vi "SO2 43i Serial Data Recording & DECADEv4.0.vi"() -> ()   [LabVIEW 2014]
uses:
  <vilib>/Instr/_visa.llb/VISA Set IO Buffer Mask.ctl
  <vilib>/Platform/TimedLoop/XDataNode/timing_clust.ctl
  <vilib>/Platform/TimedLoop/XDataNode/nitl_modes.ctl
  <vilib>/Platform/TimedLoop/XDataNode/wakeup.ctl
  C:/Program Files (x86)/National Instruments/LabVIEW 2014/examples/Data Communication/Network Streams/Simple Network Streams/support/Network Stream Command.ctl
  <vilib>/Utility/error.llb/whitespace.ctl
  <vilib>/Instr/_visa.llb/VISA Configure Serial Port (Instr).vi
  <vilib>/Utility/file.llb/Read From Spreadsheet File (string).vi
  <vilib>/Utility/tcp.llb/UDP Multicast Write-Only Open.vi
  <vilib>/platform/TimedLoop/XDataNode/XDataNode.xnode
  <vilib>/Platform/TimedLoop/XDataNode/XDNodeRunTimeDep.lvlib
  <vilib>/ptbypt/NI_PtbyPt.lvlib
panel:
  out "local\ndummy":bool
  out "cal gas cylinder conc":dbl=500.0 format="%.4g"
  out "calcon save to file":bool
  out "ev8 zero interval":i32=600
  out "Auto Zeroing":bool
  out "Simulate MOCCA Conc":dbl
  out "MOCCA window delay time (sec)":i32=30
  out "MOCCA SO2 Limit":i32=800
  out "SO2 Inflight MOCCA Alarm\n(default = OFF)":bool
  out "ev8 user set time":i32=60
  out "Mean Cal Offset":dbl
  out "Mean Cal\n(default = ON)":bool=TRUE
  out "Default file name":string
  out "Stop File Write":bool
  out "error out 4":errorcluster
  out "V6":bool
  out "V8":bool
  out "V9":bool
  out "error out 2":errorcluster
  in  "MFC_2 SLPM set value":dbl
  out "Value Read 2":string
  out "status 2":bool
  out "MFC 2":dbl[](array[numeric])
  in  "VISA resource name 3":refnum<visa-resource-name>="ASRL4::INSTR"
  in  "timeout (10sec) 3":u32=3000
  out "error out 3":errorcluster
  in  "MFC_3 SLPM set value":dbl=2.0
  out "Value Read 3":string
  out "status":bool
  out "MFC 3":dbl[](array[numeric])
  in  "VISA resource name 2":refnum<visa-resource-name>="ASRL5::INSTR"
  in  "timeout (10sec) 2":u32=3000
  out "Data Array UDP":string[](array[string])
  out "Slope":dbl=1.1
  out "Zero":dbl
  out "Simulate TWA Conc":dbl
  out "8hr_TWA_limit":i32=490
  out "10mins_STEL_limit":i32=800
  out "Simulate STEL Conc":dbl
  out "Simulate\nconc":bool
  out "q_size 2":i32
  out "8hr_so2_avg 2":dbl=1.0
  out "10min_so2_avg":dbl=1.0
  out "q_size":i32
  in  "Clear Display\nErrors":bool
  out "Data Processing":bool
  out "Serial Visa Error":errorcluster
  out "SEPTIC TCP Error Out":errorcluster
  out "TCP packet\nSend to SEPTIC":bool
  out "UDP Time Stamp Offset":i32=1
  out "Data Array TCP":string[](array[string])
  out "UDP packet \nstatus":bool
  out "UDP_Out_Error":errorcluster
  out "FISH TCP Error Out":errorcluster
  out "TCP packet\nSend to FISH":bool
  out "TCP Binary Packet":string
  out "Scan from String Error Counter\nfrom process loop":i32
  out "Read Error Counter\nfrom process loop":i32
  in  "milliseconds to wait":u32=330
  in  "ID":string="µ"
  in  "VISA resource name":refnum<visa-resource-name>="ASRL6::INSTR"
  out "Data In Array":string[](array[string])
  out "UDP_ASCII_Out":string
  out "UDP_Pack_num":u32
  out "Flight Number":string
  in  "dummy":string="00"
  out "Data String":string
  out "Internal packet":string[](array[string])
  out "RAW DATA":string
  in  "stop":bool
  out "Time taken history":u32(graph)
  out "Max Acq Time diff":u32
  out "Acq Time":u32
  out "Number of Send & Read Error\nfrom Acquire Loop":i32
  out "Command In":string
  # "SO2_conc"
  # "PMT_Volt"
  # "Lamp_Volt"
  # "Lamp_Intensity_Hz"
  # "Internal_Temp_degC"
  # "Reaction_Chamber_Temp_degC"
  # "Reaction_Chamber_Press_mmHg"
  # "Sample_Flow_litre_per_minute"
  # "Flag"
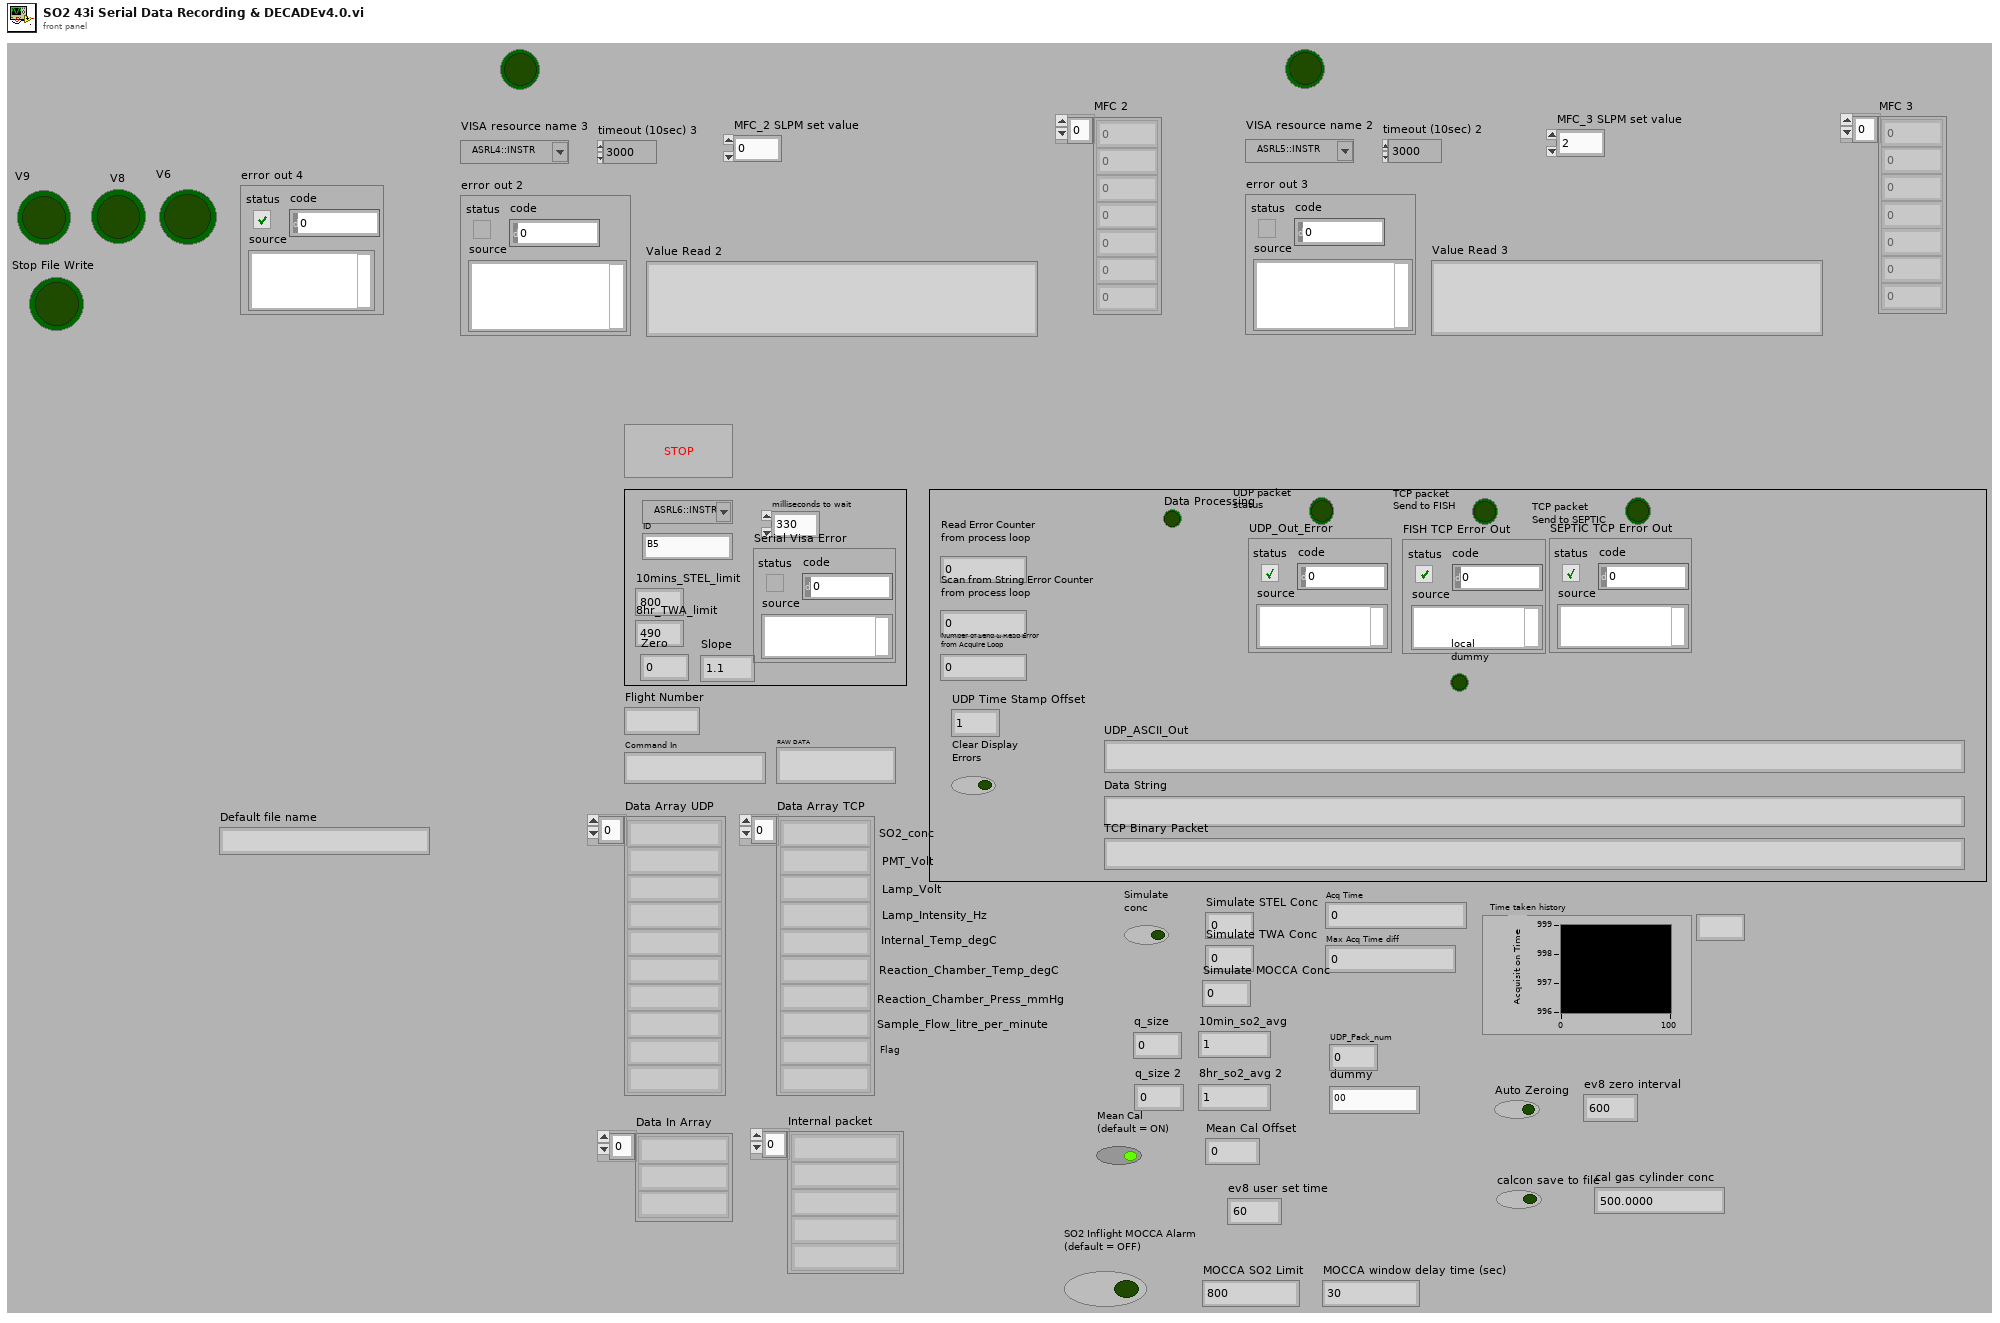
[diagram p1: front panel]
types:
  T1 = typedef "VISA Set IO Buffer Mask.ctl" = u16
  T2 = enum16{"open", "replace", "create", "open or create", "replace or create", "replace or create with confirmation"}
  T3 = typedef "Network Stream Command.ctl" = cluster{"Message":string, "Message Data":variant}
  T4 = typedef "XDNodeRunTimeDep.lvlib/timing_clust.ctl" = cluster{"Expected End [f-1]":u64, "Actual End [f-1]":u64, "Finished Late? [f-1]":bool, "Expected End [i-1]":u64, "Actual End [i-1]":u64, "Finished Late? [i-1]":bool, "Expected Start [i]":u64, "Actual Start [i]":u64, "Expected Start [f]":u64, "Actual Start [f]":u64, "Source Name":string, "Structure Name":string, "Period":i64, "Deadline":i64, "Offset":i64, "Start":i64, "Priority":i32, "Timeout":i32, "Mode":T5, "Wakeup Reason":T6, "Error":errorcluster, "Source Type":string, "Secondary Source Type":string, "Global End Time":u64, "Global Start Time":u64, "Frame Duration":u64, "Iteration Duration":u64, "Assigned CPU":i32, "I/O Scan Engine Mode":u32}
  T5 = typedef "XDNodeRunTimeDep.lvlib/nitl_modes.ctl" = enum32{"No Change", "Process missed periods, maintain original phase", "Discard missed periods, maintain original phase", "Process missed periods, ignore original phase", "Discard missed periods, ignore original phase"}
  T6 = typedef "XDNodeRunTimeDep.lvlib/wakeup.ctl" = enum32{"Normal", "Aborted", "Asynchronous wakeup", "Timing source error", "Timed loop error", "Timeout"}
  T7 = typedef "whitespace.ctl" = u16
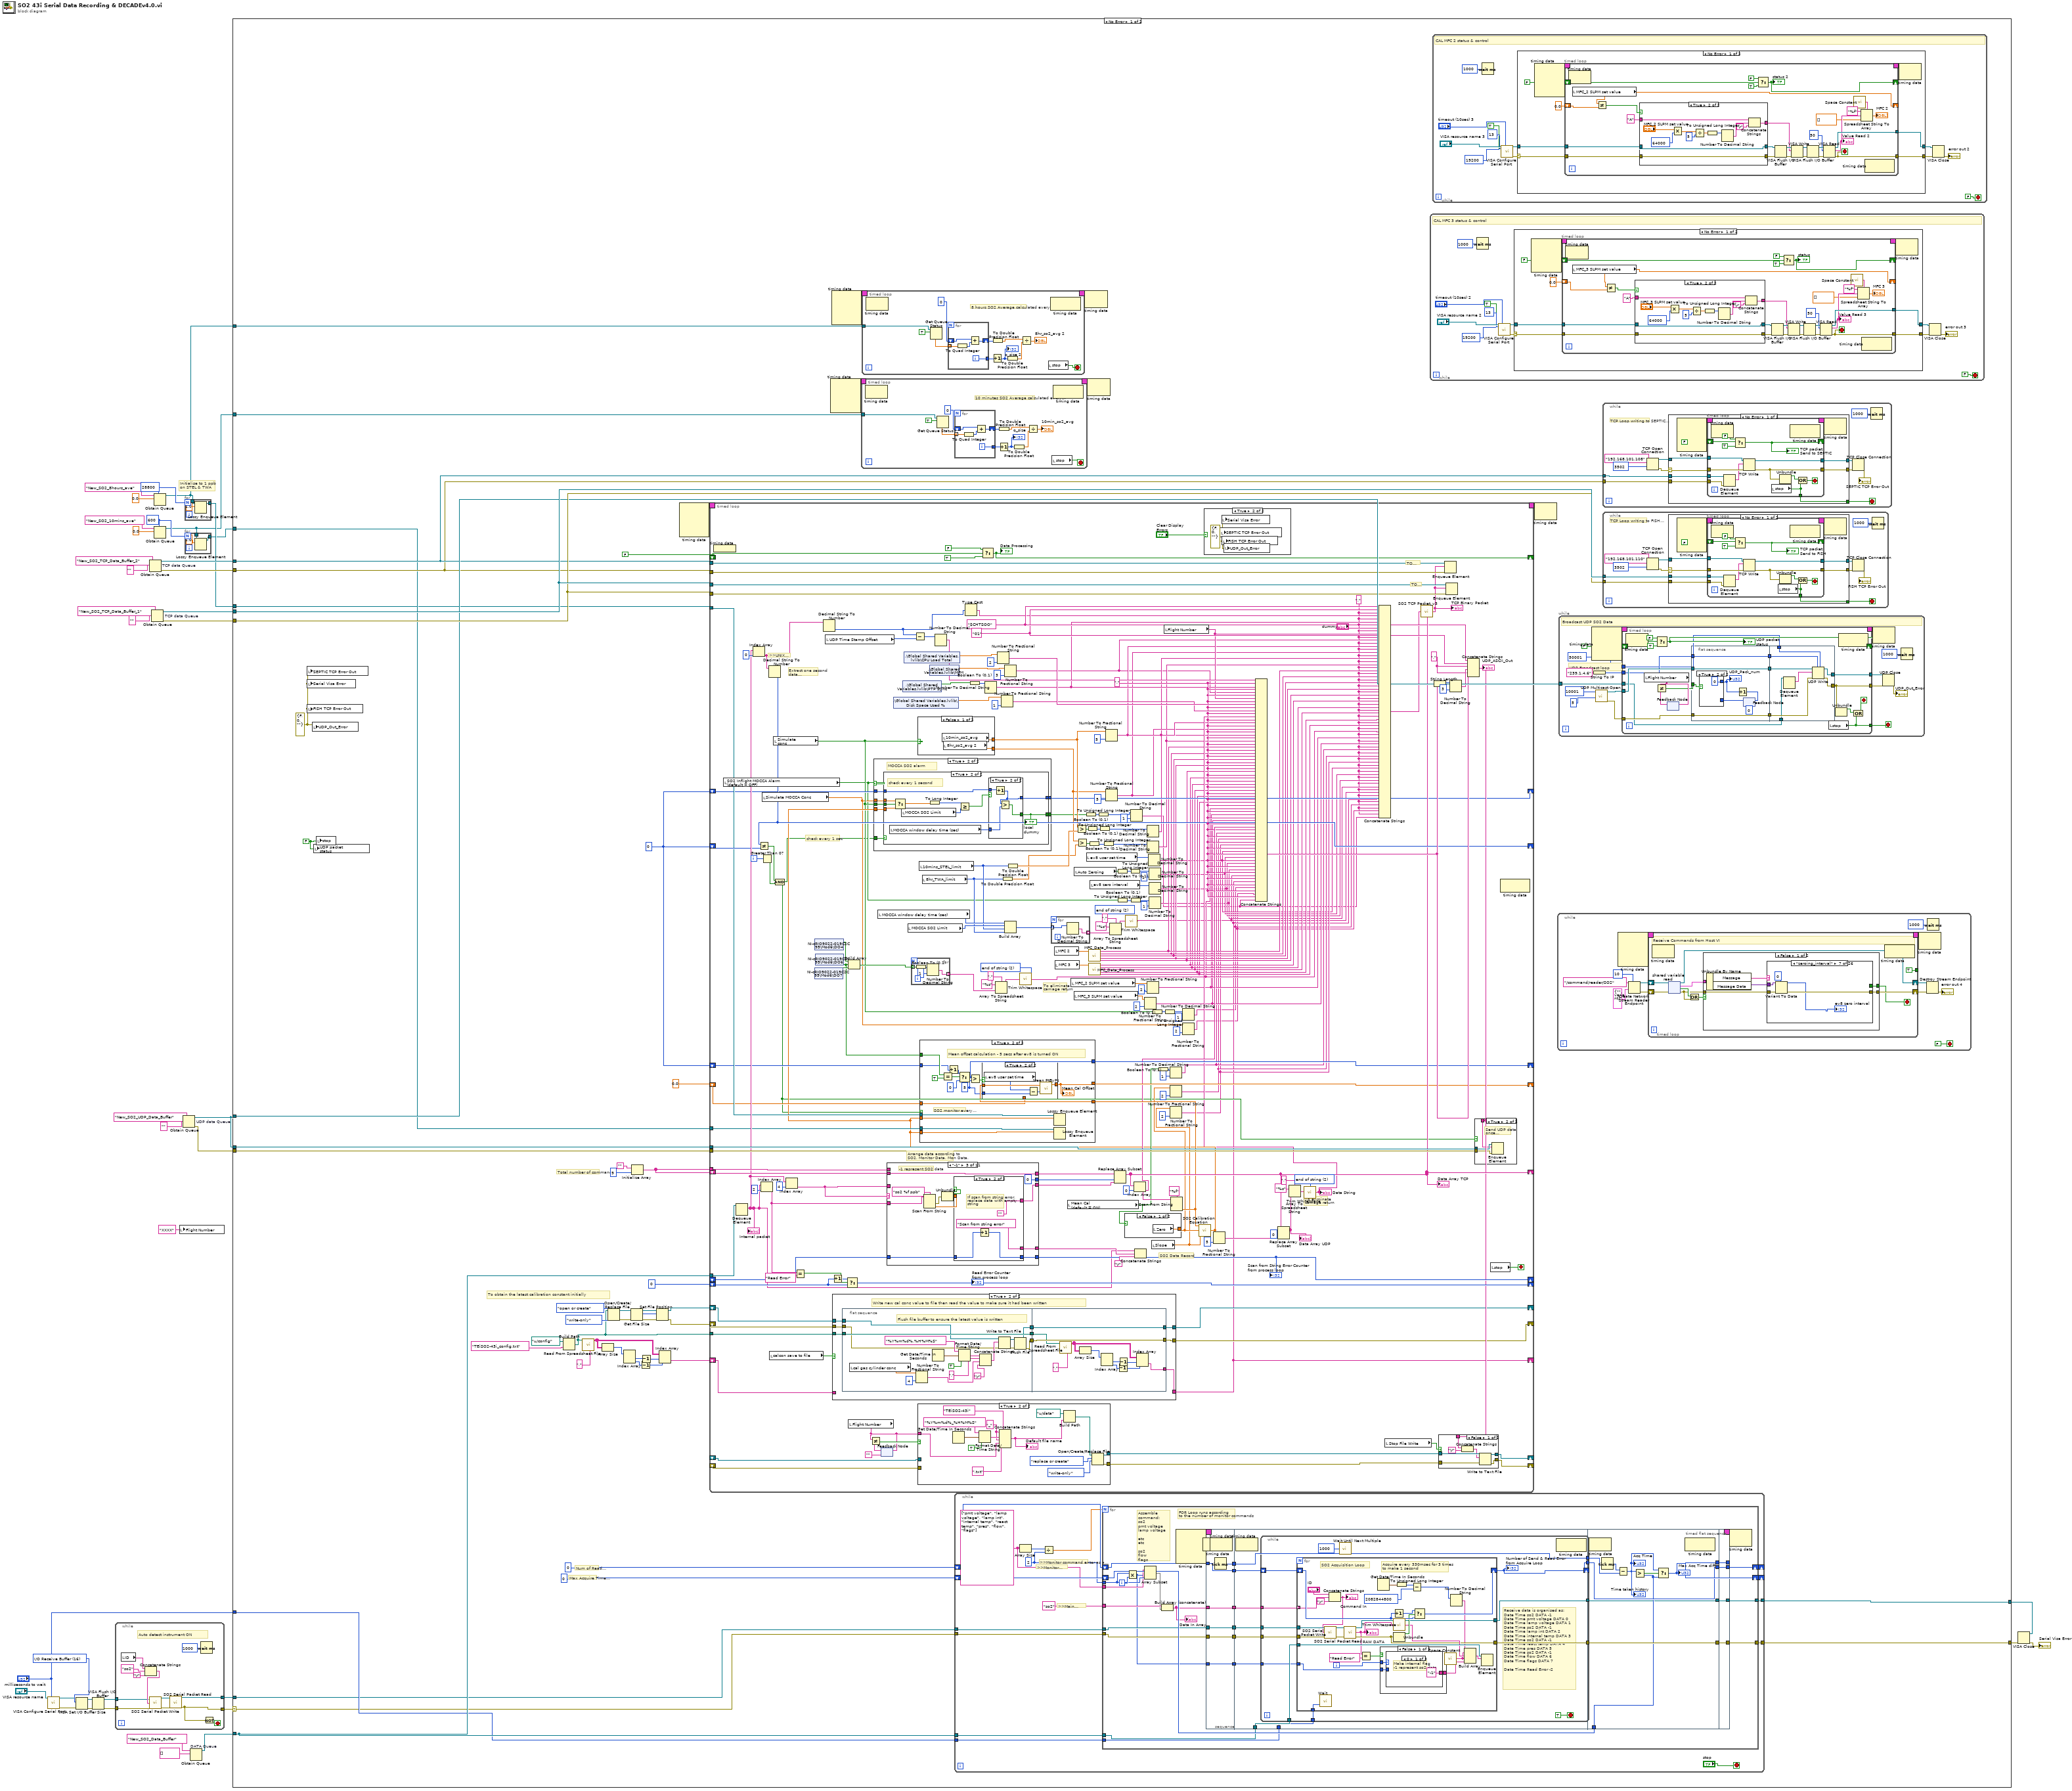
[diagram p0: block diagram]
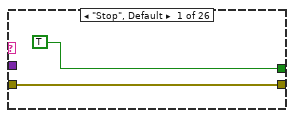
[diagram p2: hidden frame]
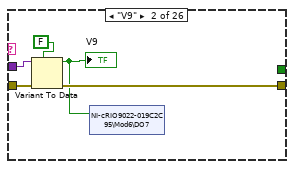
[diagram p3: hidden frame]
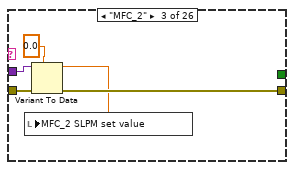
[diagram p4: hidden frame]
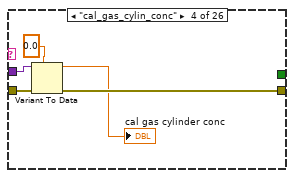
[diagram p5: hidden frame]
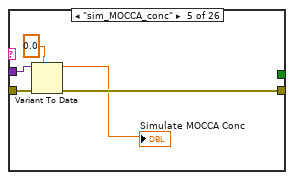
[diagram p6: hidden frame]
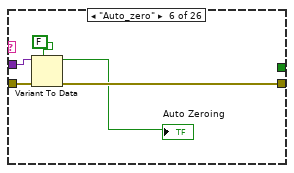
[diagram p7: hidden frame]
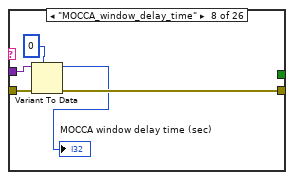
[diagram p8: hidden frame]
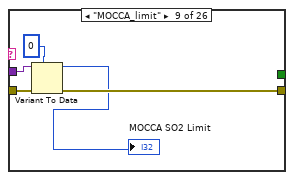
[diagram p9: hidden frame]
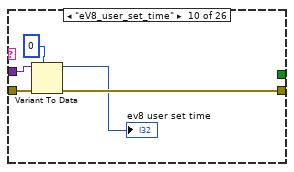
[diagram p10: hidden frame]
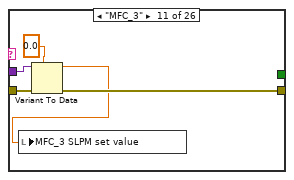
[diagram p11: hidden frame]
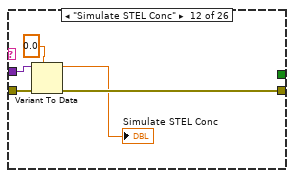
[diagram p12: hidden frame]
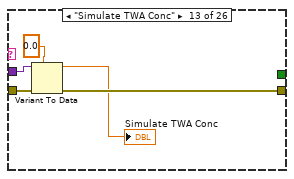
[diagram p13: hidden frame]
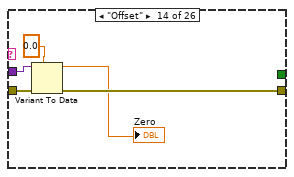
[diagram p14: hidden frame]
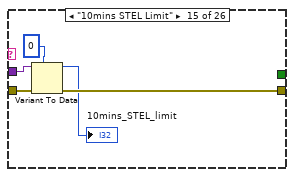
[diagram p15: hidden frame]
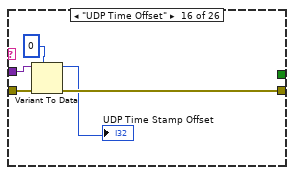
[diagram p16: hidden frame]
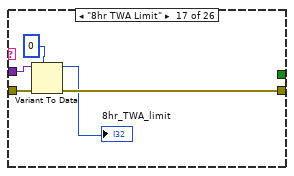
[diagram p17: hidden frame]
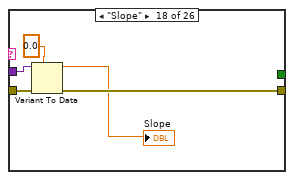
[diagram p18: hidden frame]
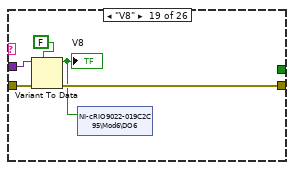
[diagram p19: hidden frame]
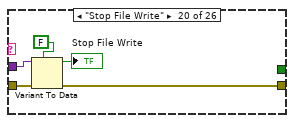
[diagram p20: hidden frame]
diagram:
  w9 = T1 16 items=["I/O Receive Buffer"=16, "I/O Transmit Buffer"=32, "I/O Receive and Transmit Buffer"=48] ("Mask")
  w16 = 28800 ("max queue size (-1, unlimited)")
  w13 = 600 ("max queue size (-1, unlimited)")
  # "Initialise to 1 ppb\non STEL & TWA"
  n1 = call-poly "VISA Configure Serial Port"("VISA resource name"="VISA resource name", "timeout (10sec)"="milliseconds to wait") -> ("VISA resource name out"=w8:refnum<visa-resource-name>, "error out"=w7:errorcluster)  [unwired: 12 in]
  n2 = VISA Set I/O Buffer Size(VISA resource name=w8, mask (16)=w9, error in (no error)=w7) -> (VISA resource name out=w2:refnum<visa-resource-name>, error out=w10:errorcluster)  [unwired: 1 in]
  n3 = VISA Flush I/O Buffer(VISA resource name=w2, error in (no error)=w10) -> (VISA resource name out=w6:refnum<visa-resource-name>, error out=w5:errorcluster)  [unwired: 1 in]
  n4 = while {
    tunnel: w6 -> [w45]
    tunnel: w5 -> [w44]
    tunnel: [w43] -> w4
    tunnel: [w42] -> w3
    stop <- w41 stop-if-true
    # "Auto detect instrument ON"
    n5 = local read "ID"() -> (w46:string)
    n6 = Concatenate Strings(w46, "so2" ("string"), "\r") -> (w49:string)
    n7 = call "SO2 Serial Packet Write.vi"("VISA resource name In"=w45, "Data in"=w49, "error in (no error)"=w44) -> ("VISA resource name Out"=w51:refnum<visa-resource-name>, "error out"=w50:errorcluster)  [unwired: 11 in]
    n8 = call "SO2 Serial Packet Read.vi"("VISA resource In"=w51, "error in"=w50) -> ("VISA resource Out"=w42:refnum<visa-resource-name>, "error out"=w43:errorcluster)  [unwired: 11 in, 1 out]
    n9 = Wait (ms)(milliseconds to wait=u32 1000) -> ()  [unwired: 1 out]
    n10 = Not(x=w43) -> (.not. x?=w41:bool)
  }
  n11 = Obtain Queue "TCP data Queue"(name (unnamed)="New_SO2_TCP_Data_Buffer_2", element data type="") -> (queue out=w23:refnum<queue>, error out=w22:errorcluster)  [unwired: 3 in, 1 out]
  n12 = Obtain Queue "TCP data Queue"(name (unnamed)="New_SO2_TCP_Data_Buffer_1", element data type="") -> (queue out=w31:refnum<queue>, error out=w30:errorcluster)  [unwired: 3 in, 1 out]
  n13 = Obtain Queue(max queue size (-1, unlimited)=w16, name (unnamed)="New_SO2_8hours_ave", element data type=0.0 ("index")) -> (queue out=w15:refnum<queue>)  [unwired: 2 in, 2 out]
  n14 = Obtain Queue(max queue size (-1, unlimited)=w13, name (unnamed)="New_SO2_10mins_ave", element data type=0.0 ("index")) -> (queue out=w12:refnum<queue>)  [unwired: 2 in, 2 out]
  n15 = local write "Flight Number"("XXXX" ("Flight Number")) -> ()
  n16 = Obtain Queue "UDP data Queue"(name (unnamed)="New_SO2_UDP_Data_Buffer", element data type="") -> (queue out=w26:refnum<queue>, error out=w27:errorcluster)  [unwired: 3 in, 1 out]
  n17 = for {
    N: w16 -> [_]
    tunnel: w15 -> [w55]
    tunnel: [w54] -> w14
    n18 = Lossy Enqueue Element(queue=w55, element=1.0) -> (queue out=w54:refnum<queue>)  [unwired: 1 in, 3 out]
  }
  n19 = for {
    N: w13 -> [_]
    tunnel: [w58] -> w11
    tunnel: w12 -> [w56]
    n20 = Lossy Enqueue Element(queue=w56, element=1.0) -> (queue out=w58:refnum<queue>)  [unwired: 1 in, 3 out]
  }
  n21 = Obtain Queue "DATA Queue"(name (unnamed)="New_SO2_Data_Buffer", element data type=string[] []) -> (queue out=w38:refnum<queue>)  [unwired: 3 in, 2 out]
  n22 = case shown="No Error" w4 {
    selector: w4 -> [w81 w1283]
    tunnel: [w112 w1283] -> w35
    tunnel: [w111 w1282] -> w36
    tunnel: w38 -> [w108 _]
    tunnel: w3 -> [w82 w1282]
    tunnel: w31 -> [w100 _]
    tunnel: w30 -> [w99 _]
    tunnel: w26 -> [w98 _]
    tunnel: w27 -> [w97 _]
    tunnel: w26 -> [w96 _]
    tunnel: w23 -> [w95 _]
    tunnel: w22 -> [w94 _]
    tunnel: "milliseconds to wait" -> [w93 _]
    tunnel: w12 -> [w90 _]
    tunnel: w15 -> [w89 _]
    tunnel: w11 -> [w88 _]
    tunnel: w14 -> [w87 _]
    frame No Error {
      w79 = 0
      w91 = errorcluster {"status"=FALSE, "code"=0, "source"=""} ("UDP Error Out")
      w102 = 0
      w101 = FALSE ("stop")
      # "To obtain the latest calibration constant initially"
      # "Max Acquire Time Diff"
      # "Num of Read Error"
      # "Total number of commands"
      n23 = local write "SEPTIC TCP Error Out"(w91) -> ()
      n24 = local write "Serial Visa Error"(w91) -> ()
      n25 = local write "FISH TCP Error Out"(w91) -> ()
      n26 = local write "UDP_Out_Error"(w91) -> ()
      n27 = local write "UDP packet \nstatus"(w101) -> ()
      n28 = local write "stop"(w101) -> ()
      n29 = Build Path(base path=path "u:/config", name or relative path="TEiSO2-43i_config.txt" ("string")) -> (appended path=w61:path)
      n30 = call-poly <vilib>:"Read From Spreadsheet File.vi"("delimiter (\\t)"="," ("delimiter (\\t)"), "file path (dialog if empty)"=w61) -> ("all rows"=w70:string[][])  [unwired: 5 in, 4 out]
      n31 = Array Size(array=w70) -> (size(s)=w71:i32[])
      n32 = Open/Create/Replace File(file path (use dialog)=w61, operation (0:open)=T2."open or create", access (0:read/write)=enum16{"read/write", "read-only", "write-only"}."write-only") -> (refnum out=w63:refnum<file>, error out=w64:errorcluster)  [unwired: 3 in, 1 out]
      n33 = Index Array(array=w71) -> (element #1=w75:i32, element #2=w73:i32)  [unwired: 2 in]
      n34 = Get File Size(file=w63, error in=w64) -> (refnum out=w65:refnum<file>, size (in bytes)=w67:i64, 0:w66:errorcluster)
      n35 = Initialize Array("", 9) -> (w103:string[])
      n36 = Decrement(x=w73) -> (x-1=w72:i32)
      n37 = Decrement(x=w75) -> (x-1=w74:i32)
      n38 = Set File Position(offset (in bytes) (0)=w67, refnum=w65, error in=w66) -> (refnum out=w60:refnum<file>, error out=w59:errorcluster)  [unwired: 1 in]
      n39 = Index Array(array=w70, index (row)=w74, index (col)=w72) -> (element=w69:string)
      n40 = node-c288() -> (w110:T4)  [unwired: 4 in]
      n41 = timed-loop {
        timing: w110 -> [_]
        timing-out: [_] -> w109
        tunnel: w108 -> [w941]
        shift-right: [w873] -> _
        shift-left: w103 -> [w931]
        shift-right: [w922] -> _
        shift-left: w102 -> [w919]
        tunnel: w103 -> [w921]
        shift-right: [w917] -> _
        shift-left: w102 -> [w918]
        tunnel: w100 -> [w915]
        tunnel: w99 -> [w914]
        tunnel: w98 -> [w913]
        tunnel: w97 -> [w912]
        shift-right: [w904] -> _
        shift-left: w79 -> [w907]
        tunnel: w95 -> [w903]
        tunnel: w94 -> [w902]
        shift-right: [w895] -> _
        shift-left: FALSE -> [w898]
        tunnel: w88 -> [w892]
        tunnel: w87 -> [w891]
        shift-right: [w860] -> _
        shift-left: _ -> [w862]
        shift-right: [w859] -> _
        shift-left: _ -> [w861]
        shift-right: [w829] -> _
        shift-left: w79 -> [w831]
        shift-right: [w827] -> _
        shift-left: 0.0 -> [w828]
        shift-right: [w817] -> _
        shift-left: w79 -> [w818]
        tunnel: w61 -> [w794]
        shift-right: [w744] -> _
        shift-left: w69 -> [w793]
        shift-right: [w784] -> _
        shift-left: w60 -> [w785]
        shift-right: [w782] -> _
        shift-left: w59 -> [w783]
        i -> [w905]
        stop <- w939 stop-if-true
        w741 = ","
        (unwired) i16 1 ("width (-)")
        (unwired) T7 2 items=["both", "start of string", "end of string"] ("location (both)")
        w837 = T7 2 items=["both", "start of string", "end of string"] ("location (both)")
        w927 = T7 2 items=["both", "start of string", "end of string"] ("location (both)")
        w787 = ","
        w777 = "01"
        w933 = ","
        w778 = "$CHTSOO"
        # "check every 1 sec"
        # "To eliminate\ncarriage return"
        # "TO SEPTIC"
        # "TO FISH"
        # "Extract one second data\nfor UDP sending"
        # "Arrange data according to\nSO2, Monitor Data, Mon Data,"
        # "To eliminate\ncarriage return"
        # ">>UNIX TIME>>"
        # "SO2 Data Record"
        n42 = node-c288() -> ()  [unwired: 1 in]
        n43 = local read "SO2 Inflight MOCCA Alarm\n(default = OFF)"() -> (w780:bool)
        n44 = Dequeue Element(queue=w941) -> (element=w910:string[])  [unwired: 2 in, 3 out]
        "Internal packet" <- w910
        n45 = Index Array(array=w910, index=0) -> (element=w909:string)
        n46 = Index Array(array=w910, index=2) -> (element=w925:string)
        n47 = Greater Than 0?(x=w905) -> (x > 0?=w908:bool)
        n48 = local read "Simulate MOCCA Conc"() -> (w788:dbl)
        n49 = Decimal String To Number(string=w909) -> (number=w904:i32)  [unwired: 2 in, 1 out]
        n50 = Not Equal?(x=w904, y=w907) -> (x != y?=w906:bool)
        n51 = local read "calcon save to file"() -> (w781:bool)
        n52 = local read "Simulate\nconc"() -> (w790:bool)
        n53 = Compound Arithmetic op=AND(w906, w908) -> (w779:bool)
        n54 = Index Array(array=w910, index=4) -> (element=w894:string)
        n55 = Equal?(x=w925, y="Read Error") -> (x = y?=w923:bool)
        n56 = shared-variable "NI-cRIO9022-019C2C95\\Mod6\\DO7"() -> (w845:bool)  [unwired: 1 in, 1 out]
        n57 = shared-variable "NI-cRIO9022-019C2C95\\Mod6\\DO4"() -> (w846:bool)  [unwired: 1 in, 1 out]
        n58 = shared-variable "NI-cRIO9022-019C2C95\\Mod6\\DO6"() -> (w832:bool)  [unwired: 1 in, 1 out]
        n59 = Decimal String To Number(string=w909) -> (number=w776:i32)  [unwired: 2 in, 1 out]
        n60 = local read "UDP Time Stamp Offset"() -> (w836:i32)
        n61 = Increment(x=w919) -> (x+1=w920:i32)
        n62 = case shown="True" w781 {
          tunnel: w794 -> [_ w953]
          tunnel: [w942 w951] -> w782
          tunnel: w793 -> [w944 _]
          tunnel: [w944 w950] -> w744
          tunnel: w785 -> [w943 w948]
          tunnel: [w943 w946] -> w784
          tunnel: w783 -> [w942 w945]
          frame False {
          }
          frame True {
            # "Write new cal conc value to file then read the value to make sure it had been written"
            n63 = flat-sequence {
              tunnel: w953 -> [w961]
              tunnel: [w956] -> w952
              tunnel: [w961] -> w949
              tunnel: w948 -> [w960]
              tunnel: [w955] -> w947
              tunnel: w945 -> [w959]
              tunnel: w952 -> [w974]
              tunnel: [w974] -> w951
              tunnel: [w973] -> w950
              tunnel: w949 -> [w972]
              tunnel: w947 -> [w971]
              tunnel: [w971] -> w946
              frame #0 {
                # "Flush file buffer to ensure the latest value is written"
                n64 = local read "cal gas cylinder conc"() -> (w954:dbl)
                n65 = Number To Fractional String(number=w954, precision (6)=i16 4) -> (F-format string=w962:string)  [unwired: 2 in]
                n66 = Get Date/Time In Seconds() -> (seconds since 1Jan1904=w969:timestamp)
                n67 = Format Date/Time String(time format string (%c)="%Y%m%d%,%H%M%S", seconds (now)=w969, UTC format=TRUE) -> (date/time string=w966:string)
                n68 = Concatenate Strings(w966, "," ("string"), w962, "\r") -> (w964:string)
                n69 = Write to Text File(file (use dialog)=w960, text=w964, error in=w959) -> (refnum out=w957:refnum<file>, error out=w958:errorcluster)  [unwired: 1 in, 1 out]
                n70 = Flush File(refnum=w957, error in=w958) -> (refnum out=w955:refnum<file>, error out=w956:errorcluster)
              }
              frame #1 {
                n71 = call-poly <vilib>:"Read From Spreadsheet File.vi"("delimiter (\\t)"="," ("delimiter (\\t)"), "file path (dialog if empty)"=w972) -> ("all rows"=w975:string[][])  [unwired: 5 in, 4 out]
                n72 = Array Size(array=w975) -> (size(s)=w976:i32[])
                n73 = Index Array(array=w976) -> (element #1=w980:i32, element #2=w978:i32)  [unwired: 2 in]
                n74 = Decrement(x=w978) -> (x-1=w977:i32)
                n75 = Decrement(x=w980) -> (x-1=w979:i32)
                n76 = Index Array(array=w975, index (row)=w979, index (col)=w977) -> (element=w973:string)
              }
            }
          }
        }
        n77 = Select(t=w920, s=w923, f=w919) -> (s? t:f=w922:i32)
        "Read Error Counter\nfrom process loop" <- w922
        n78 = Build Array(w846, w832, w845) -> (w850:bool[])
        n79 = local read "Flight Number"() -> (w863:string)
        n80 = local read "MOCCA window delay time (sec)"() -> (w799:i32)
        n81 = feedback #1("" ("Flight Number")) -> (w868:string)
        n82 = Not Equal?(x=w863, y=w868) -> (x != y?=w866:bool)
        n83 = feedback-in #1(w863) -> ()
        n84 = case shown="\"-1\"" w894 {
          tunnel: w894 -> [w1081 _ _ w1117 w1138 w1159 w1181 w1203 w1225 w1247 w1269]
          tunnel: w931 -> [w1082 _ w1096 w1118 w1139 w1160 w1182 w1204 w1226 w1248 w1270]
          tunnel: w925 -> [_ _ w1093 w1113 w1134 w1156 w1178 w1200 w1222 w1244 w1266]
          tunnel: [w1082 w1085 w1096 w1118 w1139 w1160 w1182 w1204 w1226 w1248 w1270] -> w878
          tunnel: [w1079 _ 0 ("index") w1115 w1136 w1157 w1179 w1201 w1223 w1245 w1267] -> w877
          tunnel: [_ _ w1092 w1112 w1133 w1155 w1177 w1199 w1221 w1243 w1261] -> w930
          tunnel: w921 -> [_ w1085 _ _ _ _ _ _ _ _ _]
          tunnel: w918 -> [w1077 w1084 w1089 w1109 w1130 w1150 w1173 w1194 w1217 w1238 w1260]
          tunnel: [w1077 w1084 w1088 w1108 w1129 w1149 w1172 w1193 w1216 w1237 w1259] -> w917
          tunnel: ["Internal False Flag Detected" "" w1087 w1107 w1128 w1148 w1171 w1192 w1215 w1236 w1258] -> w916
          frame "False", Default {
            n85 = Decimal String To Number(string=w1081) -> (number=w1078:i32)  [unwired: 2 in, 1 out]
            n86 = Add(x=w1078, y=1) -> (x+y=w1079:i32)
          }
          frame "-2" {
            # "Read Error Detected\nMake all data as a space"
          }
          frame "-1" {
            # "-1 represent SO2 data"
            n87 = Scan From String(format string="so2 %f ppb", input string=w1093) -> (error out=w1091:errorcluster, output 1=w1086:dbl)  [unwired: 3 in, 2 out]
            n88 = Unbundle(w1091) -> ("status"=w1090:bool)  [unwired: 2 out]
            n89 = case shown="True" w1090 {
              tunnel: w1086 -> [w1097 _]
              tunnel: [w1101 ""] -> w1092
              tunnel: w1089 -> [w1100 w1105]
              tunnel: [w1100 w1104] -> w1088
              tunnel: ["" "Scan from string error"] -> w1087
              frame False {
                # "Extract the concentration\nvalue & fixed format"
                n90 = Number To Fractional String(number=w1097, precision (6)=i16 5) -> (F-format string=w1101:string)  [unwired: 2 in]
              }
              frame True {
                # "If scan from string error,\nreplace data with empty\nstring"
                n91 = Increment(x=w1105) -> (x+1=w1104:i32)
              }
            }
          }
          frame "0" {
            # "0 represents pmt voltage -0510 volts"
            n92 = Scan From String(format string="pmt voltage %d", input string=w1113) -> (error out=w1111:errorcluster, output 1=w1106:i32)  [unwired: 3 in, 2 out]
            n93 = Decimal String To Number(string=w1117) -> (number=w1116:i32)  [unwired: 2 in, 1 out]
            n94 = Unbundle(w1111) -> ("status"=w1110:bool)  [unwired: 2 out]
            n95 = case shown="False" w1110 {
              tunnel: w1106 -> [w1122 _]
              tunnel: [w1119 w1123] -> w1112
              tunnel: w1109 -> [w1121 w1126]
              tunnel: [w1121 w1125] -> w1108
              tunnel: ["" "Scan from string error"] -> w1107
              tunnel: [w1119 w1123] -> _
              frame False {
                # "Extract the actual value\n& fixed format"
                n96 = Number To Decimal String(number=w1122) -> (decimal integer string=w1119:string)  [unwired: 1 in]
              }
              frame True {
                w1123 = ""
                # "If scan from string error,\nreplace data with empty\nstring"
                n97 = Increment(x=w1126) -> (x+1=w1125:i32)
              }
            }
            n98 = Increment(x=w1116) -> (x+1=w1115:i32)
          }
          frame "1" {
            # "1 represents lamp voltage; lamp voltage 810 volts"
            n99 = Scan From String(format string="lamp voltage %d", input string=w1134) -> (error out=w1132:errorcluster, output 1=w1127:i32)  [unwired: 3 in, 2 out]
            n100 = Decimal String To Number(string=w1138) -> (number=w1137:i32)  [unwired: 2 in, 1 out]
            n101 = Unbundle(w1132) -> ("status"=w1131:bool)  [unwired: 2 out]
            n102 = case shown="True" w1131 {
              tunnel: w1127 -> [w1143 _]
              tunnel: [w1140 w1144] -> w1133
              tunnel: w1130 -> [w1142 w1147]
              tunnel: [w1142 w1146] -> w1129
              tunnel: ["" "Scan from string error"] -> w1128
              tunnel: [w1140 w1144] -> _
              frame False {
                # "Extract the actual value\n& fixed format"
                n103 = Number To Decimal String(number=w1143) -> (decimal integer string=w1140:string)  [unwired: 1 in]
              }
              frame True {
                w1144 = ""
                # "If scan from string error,\nreplace data with empty\nstring"
                n104 = Increment(x=w1147) -> (x+1=w1146:i32)
              }
            }
            n105 = Increment(x=w1137) -> (x+1=w1136:i32)
          }
          frame "2" {
            # "2 represents lamp intensity; lamp int 35867 Hz"
            n106 = Scan From String(format string="lamp int %d", input string=w1156) -> (error out=w1152:errorcluster, output 1=w1153:i32)  [unwired: 3 in, 2 out]
            n107 = Decimal String To Number(string=w1159) -> (number=w1158:i32)  [unwired: 2 in, 1 out]
            n108 = Unbundle(w1152) -> ("status"=w1151:bool)  [unwired: 2 out]
            n109 = case shown="True" w1151 {
              tunnel: [w1161 w1166] -> w1155
              tunnel: w1153 -> [w1165 _]
              tunnel: w1150 -> [w1164 w1169]
              tunnel: [w1164 w1168] -> w1149
              tunnel: ["" "Scan from string error"] -> w1148
              tunnel: [w1161 w1166] -> _
              frame False {
                # "Extract the actual value\n& fixed format"
                n110 = Number To Fractional String(number=w1165, precision (6)=i16 0) -> (F-format string=w1161:string)  [unwired: 2 in]
              }
              frame True {
                w1166 = ""
                # "If scan from string error,\nreplace data with empty\nstring"
                n111 = Increment(x=w1169) -> (x+1=w1168:i32)
              }
            }
            n112 = Increment(x=w1158) -> (x+1=w1157:i32)
          }
          frame "3" {
            # "3 represents internal temp; internal temp 027.2 deg C, actual 027.2"
            n113 = Scan From String(format string="%[^,], %s %f", input string=w1178) -> (error out=w1175:errorcluster, output 3=w1170:dbl)  [unwired: 7 in, 2 out]
            n114 = Decimal String To Number(string=w1181) -> (number=w1180:i32)  [unwired: 2 in, 1 out]
            n115 = Unbundle(w1175) -> ("status"=w1174:bool)  [unwired: 2 out]
            n116 = case shown="True" w1174 {
              tunnel: [w1183 w1188] -> w1177
              tunnel: w1170 -> [w1187 _]
              tunnel: w1173 -> [w1186 w1191]
              tunnel: [w1186 w1190] -> w1172
              tunnel: ["" "Scan from string error"] -> w1171
              tunnel: [w1183 w1188] -> _
              frame False {
                # "Extract the actual value\n& fixed format"
                n117 = Number To Fractional String(number=w1187, precision (6)=i16 1) -> (F-format string=w1183:string)  [unwired: 2 in]
              }
              frame True {
                w1188 = ""
                # "If scan from string error,\nreplace data with empty\nstring"
                n118 = Increment(x=w1191) -> (x+1=w1190:i32)
              }
            }
            n119 = Increment(x=w1180) -> (x+1=w1179:i32)
          }
          frame "4" {
            # "4 represents react temp; react temp 045.2 deg C"
            n120 = Scan From String(format string="react temp %f deg C", input string=w1200) -> (error out=w1196:errorcluster, output 1=w1197:dbl)  [unwired: 3 in, 2 out]
            n121 = Decimal String To Number(string=w1203) -> (number=w1202:i32)  [unwired: 2 in, 1 out]
            n122 = Unbundle(w1196) -> ("status"=w1195:bool)  [unwired: 2 out]
            n123 = case shown="False" w1195 {
              tunnel: [w1205 w1210] -> w1199
              tunnel: w1197 -> [w1209 _]
              tunnel: w1194 -> [w1208 w1213]
              tunnel: [w1208 w1212] -> w1193
              tunnel: ["" "Scan from string error"] -> w1192
              tunnel: [w1205 w1210] -> _
              frame False {
                # "Extract the actual value\n& fixed format"
                n124 = Number To Fractional String(number=w1209, precision (6)=i16 1) -> (F-format string=w1205:string)  [unwired: 2 in]
              }
              frame True {
                w1210 = ""
                # "If scan from string error,\nreplace data with empty\nstring"
                n125 = Increment(x=w1213) -> (x+1=w1212:i32)
              }
            }
            n126 = Increment(x=w1202) -> (x+1=w1201:i32)
          }
          frame "5" {
            # "5 represents chamber pressure; pres 760.0 mm Hg, actual 753.4"
            n127 = Scan From String(format string="%[^,], %s %f", input string=w1222) -> (error out=w1219:errorcluster, output 3=w1214:dbl)  [unwired: 7 in, 2 out]
            n128 = Decimal String To Number(string=w1225) -> (number=w1224:i32)  [unwired: 2 in, 1 out]
            n129 = Unbundle(w1219) -> ("status"=w1218:bool)  [unwired: 2 out]
            n130 = case shown="False" w1218 {
              tunnel: [w1227 w1232] -> w1221
              tunnel: w1214 -> [w1231 _]
              tunnel: w1217 -> [w1230 w1235]
              tunnel: [w1230 w1234] -> w1216
              tunnel: ["" "Scan from string error"] -> w1215
              tunnel: [w1227 w1232] -> _
              frame False {
                # "Extract the actual value\n& fixed format"
                n131 = Number To Fractional String(number=w1231, precision (6)=i16 1) -> (F-format string=w1227:string)  [unwired: 2 in]
              }
              frame True {
                w1232 = ""
                # "If scan from string error,\nreplace data with empty\nstring"
                n132 = Increment(x=w1235) -> (x+1=w1234:i32)
              }
            }
            n133 = Increment(x=w1224) -> (x+1=w1223:i32)
          }
          frame "6" {
            # "6 represents flow data; flow 0.503 l/m"
            n134 = Scan From String(format string="flow %f l/m", input string=w1244) -> (error out=w1240:errorcluster, output 1=w1241:dbl)  [unwired: 3 in, 2 out]
            n135 = Decimal String To Number(string=w1247) -> (number=w1246:i32)  [unwired: 2 in, 1 out]
            n136 = Unbundle(w1240) -> ("status"=w1239:bool)  [unwired: 2 out]
            n137 = case shown="True" w1239 {
              tunnel: [w1253 ""] -> w1243
              tunnel: w1241 -> [w1252 _]
              tunnel: w1238 -> [w1251 w1256]
              tunnel: [w1251 w1255] -> w1237
              tunnel: ["" "Scan from string error"] -> w1236
              frame False {
                # "Extract the actual value\n& fixed format"
                n138 = Number To Fractional String(number=w1252, precision (6)=i16 3) -> (F-format string=w1253:string)  [unwired: 2 in]
              }
              frame True {
                # "If scan from string error,\nreplace data with empty\nstring"
                n139 = Increment(x=w1256) -> (x+1=w1255:i32)
              }
            }
            n140 = Increment(x=w1246) -> (x+1=w1245:i32)
          }
          frame "7" {
            # "7 represents flags data; flags 1c100000"
            n141 = Scan From String(format string="flags %s", input string=w1266) -> (error out=w1264:errorcluster, output 1=w1262:string)  [unwired: 3 in, 2 out]
            n142 = Decimal String To Number(string=w1269) -> (number=w1268:i32)  [unwired: 2 in, 1 out]
            n143 = Unbundle(w1264) -> ("status"=w1263:bool)  [unwired: 2 out]
            n144 = case shown="False" w1263 {
              tunnel: w1262 -> [w1273 _]
              tunnel: [w1273 ""] -> w1261
              tunnel: w1260 -> [w1272 w1276]
              tunnel: [w1272 w1275] -> w1259
              tunnel: ["" "Scan from string error"] -> w1258
              frame False {
                # "Extract the actual value\n& fixed format"
              }
              frame True {
                # "If scan from string error,\nreplace data with empty\nstring"
                n145 = Increment(x=w1276) -> (x+1=w1275:i32)
              }
            }
            n146 = Increment(x=w1268) -> (x+1=w1267:i32)
          }
        }
        "Scan from String Error Counter\nfrom process loop" <- w917
        n147 = shared-variable ".\\Global Shared Variables.lvlib\\Disk Space Used %"() -> (w839:dbl)  [unwired: 1 in, 1 out]
        n148 = shared-variable ".\\Global Shared Variables.lvlib\\PTP Sync"() -> (w852:bool)  [unwired: 1 in, 1 out]
        n149 = shared-variable ".\\Global Shared Variables.lvlib\\CPU Load Total"() -> (w856:dbl)  [unwired: 1 in, 1 out]
        n150 = local read "MOCCA SO2 Limit"() -> (w798:i32)
        n151 = for {
          tunnel: w850 -> [w1020] mode=indexing
          tunnel: [w1019] -> w847 mode=indexing
          n152 = Boolean To (0,1)(Boolean=w1020) -> (0, 1=w1021:i16)
          n153 = Number To Decimal String(number=w1021, width (-)=i16 1) -> (decimal integer string=w1019:string)
        }
        n154 = Subtract(x=w776, y=w836) -> (x-y=w900:i32)
        n155 = case shown="False" w790 {
          tunnel: [w1013 w1014] -> w887
          tunnel: [w1012 w1015] -> w885
          frame False {
            n156 = local read "10min_so2_avg"() -> (w1013:dbl)
            n157 = local read "8hr_so2_avg 2"() -> (w1012:dbl)
          }
          frame True {
            # "SO2 STEL & TWA simulate"
            n158 = local read "Simulate STEL Conc"() -> (w1014:dbl)
            n159 = local read "Simulate TWA Conc"() -> (w1015:dbl)
          }
        }
        n160 = case shown="True" w866 {
          tunnel: [w1023 w1026] -> w865
          tunnel: [w1022 w1025] -> w864
          tunnel: w862 -> [w1023 _]
          tunnel: w861 -> [w1022 _]
          tunnel: w863 -> [_ w1024]
          frame False {
          }
          frame True {
            w1033 = "_" ("string")
            n161 = Get Date/Time In Seconds() -> (seconds since 1Jan1904=w1034:timestamp)
            n162 = Format Date/Time String(time format string (%c)="%Y%m%d%_%H%M%S", seconds (now)=w1034, UTC format=TRUE) -> (date/time string=w1037:string)
            n163 = Concatenate Strings("TEiSO2-43i" ("string"), w1033, w1037, w1033, w1024, ".txt" ("string")) -> (w1031:string)
            "Default file name" <- w1031
            n164 = Build Path(base path=path "u:/data", name or relative path=w1031) -> (appended path=w1027:path)
            n165 = Open/Create/Replace File(file path (use dialog)=w1027, operation (0:open)=T2."replace or create", access (0:read/write)=enum16{"read/write", "read-only", "write-only"}."write-only") -> (refnum out=w1026:refnum<file>, error out=w1025:errorcluster)  [unwired: 3 in, 1 out]
          }
        }
        n166 = local read "10mins_STEL_limit"() -> (w797:i32)
        n167 = local read "8hr_TWA_limit"() -> (w796:i32)
        n168 = shared-variable ".\\Global Shared Variables.lvlib\\MFM"() -> (w853:dbl)  [unwired: 1 in, 1 out]
        n169 = Number To Decimal String(number=w900) -> (decimal integer string=w899:string)  [unwired: 1 in]
        n170 = Type Cast(x=w776) -> (*(type *) &x=w775:string)  [unwired: 1 in]
        n171 = Boolean To (0,1)(Boolean=w852) -> (0, 1=w851:i16)
        n172 = Select(t=FALSE, s=w898, f=TRUE) -> (s? t:f=w895:bool)
        "Data Processing" <- w895
        n173 = Number To Decimal String(number=w851) -> (decimal integer string=w774:string)  [unwired: 1 in]
        n174 = Array To Spreadsheet String(delimiter (Tab)=",", array=w847, 3:"%s" ("format string")) -> (spreadsheet string=w838:string)
        n175 = Number To Fractional String(number=w856, precision (6)=i16 2) -> (F-format string=w835:string)  [unwired: 2 in]
        n176 = Number To Fractional String(number=w839, precision (6)=i16 1) -> (F-format string=w834:string)  [unwired: 2 in]
        n177 = To Double Precision Float(number=w796) -> (double precision float=w888:dbl)
        n178 = Number To Fractional String(number=w853, precision (6)=i16 3) -> (F-format string=w766:string)  [unwired: 2 in]
        n179 = Build Array(w799, w798, w797, w796) -> (w795:i32[])
        n180 = To Double Precision Float(number=w797) -> (double precision float=w889:dbl)
        n181 = call <vilib>:"Trim Whitespace.vi"("string"=w838, "location (both)"=w837) -> ("trimmed string"=w755:string)
        n182 = for {
          tunnel: w795 -> [w982] mode=indexing
          tunnel: [w983] -> w801 mode=indexing
          n183 = Number To Decimal String(number=w982) -> (decimal integer string=w983:string)  [unwired: 1 in]
        }
        n184 = local read "MFC 2"() -> (w870:dbl[])
        n185 = local read "MFC 3"() -> (w869:dbl[])
        n186 = local read "Mean Cal\n(default = ON)"() -> (w823:bool)
        n187 = local read "MFC_2 SLPM set value"() -> (w842:dbl)
        n188 = local read "MFC_3 SLPM set value"() -> (w841:dbl)
        n189 = local read "Auto Zeroing"() -> (w809:bool)
        n190 = Greater?(x=w887, y=w889) -> (0:w882:bool)
        n191 = Greater?(x=w885, y=w888) -> (0:w881:bool)
        n192 = local read "ev8 user set time"() -> (w812:i32)
        n193 = Boolean To (0,1)(Boolean=w882) -> (0, 1=w884:i16)
        n194 = Boolean To (0,1)(Boolean=w881) -> (0, 1=w883:i16)
        n195 = call "MFC_Data_Process.vi"("MFC"=w870) -> ("MFC Absolute Pressure"=w765:string, "MFC Temperature"=w764:string, "MFC Volumetric Flow"=w763:string, "MFC Mass Flow"=w762:string, "MFC Set Point"=w761:string)  [unwired: 10 in]
        n196 = call "MFC_Data_Process.vi"("MFC"=w869) -> ("MFC Absolute Pressure"=w760:string, "MFC Temperature"=w759:string, "MFC Volumetric Flow"=w758:string, "MFC Mass Flow"=w757:string, "MFC Set Point"=w756:string)  [unwired: 10 in]
        n197 = local read "ev8 zero interval"() -> (w808:i32)
        n198 = To Unsigned Long Integer(number=w884) -> (unsigned 32bit integer=w880:u32)
        n199 = To Unsigned Long Integer(number=w883) -> (unsigned 32bit integer=w879:u32)
        n200 = Number To Fractional String(number=w887, precision (6)=i16 5) -> (F-format string=w770:string)  [unwired: 2 in]
        n201 = Number To Fractional String(number=w885, precision (6)=i16 5) -> (F-format string=w769:string)  [unwired: 2 in]
        n202 = Array To Spreadsheet String(delimiter (Tab)=",", array=w801, 3:"%s" ("format string")) -> (spreadsheet string=w800:string)
        n203 = Replace Array Subset(array=w878, new element=w930, index=w877) -> (w873:string[])
        "Data Array TCP" <- w873
        n204 = Boolean To (0,1)(Boolean=w809) -> (0, 1=w811:i16)
        n205 = Boolean To (0,1)(Boolean=w780) -> (0, 1=w807:i16)
        n206 = case shown="False" w823 {
          tunnel: [w1016 w1017] -> w820
          frame False {
            n207 = local read "Zero"() -> (w1016:dbl)
          }
          frame True {
            n208 = local read "Mean Cal Offset"() -> (w1017:dbl)
          }
        }
        n209 = call <vilib>:"Trim Whitespace.vi"("string"=w800) -> ("trimmed string"=w745:string)  [unwired: 1 in]
        n210 = To Unsigned Long Integer(number=w811) -> (unsigned 32bit integer=w810:u32)
        n211 = To Unsigned Long Integer(number=w807) -> (unsigned 32bit integer=w806:u32)
        n212 = Index Array(array=w873, index=0) -> (element=w826:string)
        n213 = Concatenate Strings(w910, w916, "\r") -> ()  [unwired: 1 out]
        n214 = Number To Fractional String(number=w841, precision (6)=i16 2) -> (F-format string=w753:string)  [unwired: 2 in]
        n215 = Number To Decimal String(number=w880) -> (decimal integer string=w768:string)  [unwired: 1 in]
        n216 = Number To Decimal String(number=w879) -> (decimal integer string=w767:string)  [unwired: 1 in]
        n217 = Number To Fractional String(number=w842, precision (6)=i16 2) -> (F-format string=w754:string)  [unwired: 2 in]
        n218 = Number To Decimal String(number=w812) -> (decimal integer string=w749:string)  [unwired: 1 in]
        n219 = Number To Decimal String(number=w810, width (-)=i16 1) -> (decimal integer string=w748:string)
        n220 = Number To Decimal String(number=w808) -> (decimal integer string=w747:string)  [unwired: 1 in]
        n221 = Number To Decimal String(number=w806, width (-)=i16 1) -> (decimal integer string=w746:string)
        n222 = Boolean To (0,1)(Boolean=w790) -> (0, 1=w792:i16)
        n223 = local read "Slope"() -> (w819:dbl)
        n224 = Boolean To (0,1)(Boolean=w823) -> (0, 1=w825:i16)
        n225 = local read "Flight Number"() -> (w772:string)
        n226 = To Unsigned Long Integer(number=w792) -> (unsigned 32bit integer=w791:u32)
        n227 = Number To Fractional String(number=w819, precision (6)=i16 2) -> (F-format string=w750:string)  [unwired: 2 in]
        n228 = Number To Decimal String(number=w825, width (-)=i16 1) -> (decimal integer string=w752:string)
        n229 = Number To Fractional String(number=w820, precision (6)=i16 2) -> (F-format string=w751:string)  [unwired: 2 in]
        n230 = Scan From String(format string="%f", input string=w826) -> (output 1=w830:dbl)  [unwired: 3 in, 3 out]
        n231 = Number To Decimal String(number=w791) -> (decimal integer string=w743:string)  [unwired: 1 in]
        n232 = Number To Fractional String(number=w788, precision (6)=i16 2) -> (F-format string=w742:string)  [unwired: 2 in]
        n233 = call "SO2 Calibration Equation.vi"("Input"=w830, "Offset"=w820, "Slope"=w819) -> ("Output"=w816:dbl)  [unwired: 12 in]
        n234 = case shown="True" w780 {
          tunnel: w818 -> [_ w989]
          tunnel: [0 w987] -> w817
          tunnel: w790 -> [_ w992]
          tunnel: w788 -> [_ w991]
          tunnel: w816 -> [_ w990]
          tunnel: [FALSE w988] -> w813
          tunnel: w779 -> [_ w986]
          frame False {
          }
          frame True {
            # "MOCCA SO2 alarm"
            n235 = case shown="True" w986 {
              tunnel: w992 -> [_ w1002]
              tunnel: w991 -> [_ w1001]
              tunnel: w990 -> [_ w1000]
              tunnel: w989 -> [w994 w999]
              tunnel: [w993 w997] -> w988
              tunnel: [w994 w996] -> w987
              frame False {
                n236 = local read "local\ndummy"() -> (w993:bool)
              }
              frame True {
                # "check every 1 second"
                n237 = local read "MOCCA window delay time (sec)"() -> (w998:i32)
                n238 = Select(t=w1001, s=w1002, f=w1000) -> (s? t:f=w1003:dbl)
                n239 = local read "MOCCA SO2 Limit"() -> (w1004:i32)
                n240 = To Long Integer(number=w1003) -> (32bit integer=w1005:i32)
                n241 = Greater Or Equal?(x=w1005, y=w1004) -> (x >= y?=w995:bool)
                n242 = case shown="True" w995 {
                  tunnel: w999 -> [_ w1011]
                  tunnel: w998 -> [_ w1010]
                  tunnel: [FALSE w1009] -> w997
                  tunnel: [0 w1008] -> w996
                  frame False {
                  }
                  frame True {
                    n243 = Increment(x=w1011) -> (x+1=w1008:i32)
                    n244 = Greater?(x=w1008, y=w1010) -> (0:w1009:bool)
                  }
                }
                "local\ndummy" <- w997
              }
            }
          }
        }
        n245 = case shown="True" w779 {
          tunnel: w892 -> [_ w1065]
          tunnel: w816 -> [_ w1062]
          tunnel: w816 -> [_ w1064]
          tunnel: w891 -> [_ w1063]
          tunnel: w832 -> [_ w1058]
          tunnel: w831 -> [w1049 w1057]
          tunnel: w830 -> [_ w1055]
          tunnel: [w1049 w1053] -> w829
          tunnel: w828 -> [w1048 w1052]
          tunnel: [w1048 w1051] -> w827
          frame False {
          }
          frame True {
            w1050 = 5 ("y")
            # "Mean offset calculation - 5 secs after ev8 is turned ON"
            # "SO2 monitor every second"
            n246 = Equal?(x=w1058, y=TRUE) -> (x = y?=w1060:bool)
            n247 = Increment(x=w1057) -> (x+1=w1059:i32)
            n248 = Select(t=w1059, s=w1060, f=0) -> (s? t:f=w1053:i32)
            n249 = Greater?(x=w1053, y=w1050) -> (0:w1056:bool)
            n250 = case shown="True" w1056 {
              tunnel: w1055 -> [_ w1071]
              tunnel: [w1066 w1070] -> w1051
              tunnel: w1052 -> [w1066 _]
              tunnel: w1050 -> [_ w1069]
              frame False {
              }
              frame True {
                n251 = local read "ev8 user set time"() -> (w1067:i32)
                n252 = Subtract(x=w1067, y=w1069) -> (x-y=w1068:i32)
                n253 = call <vilib>:"Mean PtByPt.vi"("x"=w1071, "sample length"=w1068) -> ("mean"=w1070:dbl)  [unwired: 2 in, 1 out]
              }
            }
            "Mean Cal Offset" <- w1051
            n254 = Lossy Enqueue Element(queue=w1065, element=w1062) -> ()  [unwired: 1 in, 4 out]
            n255 = Lossy Enqueue Element(queue=w1063, element=w1064) -> ()  [unwired: 1 in, 4 out]
          }
        }
        n256 = Boolean To (0,1)(Boolean=w813) -> (0, 1=w815:i16)
        n257 = To Unsigned Long Integer(number=w815) -> (unsigned 32bit integer=w814:u32)
        n258 = Number To Decimal String(number=w814, width (-)=i16 1) -> (decimal integer string=w740:string)
        n259 = case shown="True" "Clear Display\nErrors" {
          frame False {
          }
          frame True {
            w1072 = errorcluster {"status"=FALSE, "code"=0, "source"=""} ("UDP Error Out")
            n260 = local write "SEPTIC TCP Error Out"(w1072) -> ()
            n261 = local write "Serial Visa Error"(w1072) -> ()
            n262 = local write "FISH TCP Error Out"(w1072) -> ()
            n263 = local write "UDP_Out_Error"(w1072) -> ()
          }
        }
        n264 = Number To Fractional String(number=w816, precision (6)=i16 5) -> (F-format string=w874:string)  [unwired: 2 in]
        n265 = Replace Array Subset(array=w873, new element=w874, index=0) -> (w872:string[])
        "Data Array UDP" <- w872
        n266 = Array To Spreadsheet String(delimiter (Tab)=",", array=w872, 3:"%s" ("format string")) -> (spreadsheet string=w926:string)
        n267 = call <vilib>:"Trim Whitespace.vi"("string"=w926, "location (both)"=w927) -> ("trimmed string"=w771:string)
        "Data String" <- w771
        n268 = Concatenate Strings(w899, w787, w774, w787, w766, w787, w772, w787, w835, w787, w834, w787, w771, w787, w770, w787, w769, w787, w768, w787, w767, w787, w765, w787, w764, w787, w763, w787, w762, w787, w761, w787, w760, w787, w759, w787, w758, w787, w757, w787, w756, w787, w755, w787, w754, w787, w753, w787, w826, w787, w752, w787, w751, w787, w750, w787, w749, w787, w748, w787, w747, w787, w746, w787, w745, w787, w744, w787, w743, w787, w742, w787, w740) -> (w932:string)
        n269 = Concatenate Strings(w778, w777, w741, w775, w741, w774, w741, "dummy", w741, w772, w741, w766, w741, w770, w741, w769, w741, w768, w741, w767, w741, w765, w741, w764, w741, w763, w741, w762, w741, w761, w741, w760, w741, w759, w741, w758, w741, w757, w741, w756, w741, w755, w741, w754, w741, w753, w741, w752, w741, w751, w741, w750, w741, w749, w741, w748, w741, w747, w741, w746, w741, w745, w741, w744, w741, w743, w741, w742, w741, w740) -> (w739:string)
        n270 = local read "Stop File Write"() -> (w857:bool)
        n271 = call "SO2 TCP Packet_v3.vi"("TCP Packet In"=w739, "Data Array"=w873) -> ("TCP Binary Packet"=w901:string)  [unwired: 13 in]
        "TCP Binary Packet" <- w901
        n272 = String Length(string=w932) -> (length=w936:i32)
        n273 = Enqueue Element(queue=w903, element=w901, error in (no error)=w902) -> ()  [unwired: 1 in, 3 out]
        n274 = Enqueue Element(queue=w915, element=w901, error in (no error)=w914) -> ()  [unwired: 1 in, 3 out]
        n275 = Number To Decimal String(number=w936, width (-)=i16 3) -> (decimal integer string=w934:string)
        n276 = Concatenate Strings(w778, w777, w933, w934, w933, w932) -> (w858:string)
        "UDP_ASCII_Out" <- w858
        n277 = case shown="False" w857 {
          tunnel: w858 -> [w1043 _]
          tunnel: w865 -> [w1045 w1047]
          tunnel: w864 -> [w1044 w1046]
          tunnel: [w1040 _] -> w860
          tunnel: [w1039 _] -> w859
          frame False {
            n278 = Concatenate Strings(w1043, "\r") -> (w1041:string)
            n279 = Write to Text File(file (use dialog)=w1045, text=w1041, error in=w1044) -> (refnum out=w1040:refnum<file>, error out=w1039:errorcluster)  [unwired: 2 out]
          }
          frame True {
            n280 = Close File(refnum=w1047, error in=w1046) -> ()  [unwired: 2 out]
          }
        }
        n281 = case shown="True" w779 {
          tunnel: w913 -> [_ w1075]
          tunnel: w912 -> [_ w1074]
          tunnel: w858 -> [_ w1073]
          frame False {
          }
          frame True {
            # "Send UDP data once\na second"
            n282 = Enqueue Element(queue=w1075, element=w1073, error in (no error)=w1074) -> ()  [unwired: 1 in, 3 out]
          }
        }
        n283 = local read "stop"() -> (w939:bool)
        n284 = node-c288() -> ()  [unwired: 1 in, 1 out]
      }
      n285 = node-c288() -> (w84:T4)  [unwired: 4 in]
      n286 = node-c288() -> (w86:T4)  [unwired: 4 in]
      n287 = timed-loop {
        tunnel: w90 -> [w423]
        timing: w84 -> [_]
        timing-out: [_] -> w83
        stop <- w424 stop-if-true
        # "10 minutes SO2 Average calculated every second"
        n288 = node-c288() -> ()  [unwired: 1 in, 1 out]
        n289 = Get Queue Status(queue=w423, return elements? (F)=TRUE) -> (elements=w414:dbl[])  [unwired: 1 in, 7 out]
        n290 = for {
          tunnel: w414 -> [w427] mode=indexing
          tunnel: [w431] -> w420
          shift-right: [w430] -> w418
          shift-left: i64 0 -> [w429]
          i -> [w431]
          n291 = To Quad Integer(1:w427) -> (0:w428:i64)
          n292 = Add(x=w429, y=w428) -> (x+y=w430:i64)
        }
        n293 = Increment(x=w420) -> (x+1=w415:i32)
        "q_size" <- w415
        n294 = To Double Precision Float(number=w418) -> (double precision float=w416:dbl)
        n295 = To Double Precision Float(number=w415) -> (double precision float=w417:dbl)
        n296 = Divide(x=w416, y=w417) -> (x/y=→"10min_so2_avg":dbl)
        n297 = local read "stop"() -> (w424:bool)
        n298 = node-c288() -> ()  [unwired: 1 in, 1 out]
      }
      n299 = timed-loop {
        tunnel: w89 -> [w443]
        timing: w86 -> [_]
        timing-out: [_] -> w85
        stop <- w444 stop-if-true
        # "8 hours SO2 Average calculated every second"
        n300 = node-c288() -> ()  [unwired: 1 in, 1 out]
        n301 = Get Queue Status(queue=w443, return elements? (F)=TRUE) -> (elements=w440:dbl[])  [unwired: 1 in, 7 out]
        n302 = for {
          tunnel: w440 -> [w447] mode=indexing
          tunnel: [w451] -> w439
          shift-right: [w450] -> w437
          shift-left: i64 0 -> [w449]
          i -> [w451]
          n303 = To Quad Integer(1:w447) -> (0:w448:i64)
          n304 = Add(x=w449, y=w448) -> (x+y=w450:i64)
        }
        n305 = Increment(x=w439) -> (x+1=w434:i32)
        "q_size 2" <- w434
        n306 = To Double Precision Float(number=w437) -> (double precision float=w435:dbl)
        n307 = To Double Precision Float(number=w434) -> (double precision float=w436:dbl)
        n308 = Divide(x=w435, y=w436) -> (x/y=→"8hr_so2_avg 2":dbl)
        n309 = local read "stop"() -> (w444:bool)
        n310 = node-c288() -> ()  [unwired: 1 in, 1 out]
      }
      n311 = while {
        tunnel: [w598] -> w112
        tunnel: w82 -> [w611]
        tunnel: w81 -> [w610]
        tunnel: [w609] -> w111
        tunnel: w108 -> [w608]
        shift-right: [w606] -> _
        shift-left: 0 -> [w607]
        shift-right: [w604] -> _
        shift-left: u32 0 -> [w605]
        tunnel: w93 -> [w596]
        stop <- "stop" stop-if-true
        w599 = 2
        w601 = string[] ["pmt voltage", "lamp voltage", "lamp int", "internal temp", "react temp", "pres", "flow", "flags"]
        # ">>Monitor command enter as a pair>>"
        # ">>Main commands>>"
        # ">>Monitor Command>>"
        n312 = Array Size(array=w601) -> (size(s)=w602:i32)
        n313 = Divide(x=w602, y=w599) -> (x/y=w600:dbl)
        n314 = for {
          N: w600 -> [_]
          tunnel: w611 -> [w621]
          tunnel: w610 -> [w620]
          tunnel: [w630] -> w598
          shift-right: [w628] -> w606
          shift-left: w607 -> [w629]
          shift-right: [w626] -> w604
          shift-left: w605 -> [w627]
          tunnel: [w625] -> w609
          tunnel: w608 -> [w624]
          tunnel: w601 -> [w617]
          tunnel: "so2" -> [w622]
          tunnel: w599 -> [w618]
          tunnel: w596 -> [w612]
          i -> [w619]
          # "FOR Loop runs according\nto the number of monitor commands"
          # "Assemble command:\nso2\npmt voltage\nlamp voltage\n\netc\netc\n\nso2\nflow\nflags"
          n315 = Multiply(x=w618, y=w619) -> (x*y=w615:i32)
          n316 = Array Subset(array=w617, index=w615, length=w618) -> (w616:string[])
          n317 = Build Array (concatenate)(w622, w616) -> (w623:string[])
          "Data In Array" <- w623
          n318 = node-c288() -> (w614:T4)  [unwired: 4 in]
          n319 = timed-sequence {
            timing: w614 -> [_]
            timing-out: [_] -> w613
            tunnel: w629 -> [w652]
            tunnel: w623 -> [w651]
            tunnel: w621 -> [w650]
            tunnel: w620 -> [w649]
            tunnel: w615 -> [w648]
            tunnel: w624 -> [w643]
            tunnel: [w639] -> w630
            tunnel: [w637] -> w628
            tunnel: w627 -> [w635]
            tunnel: [w634] -> w626
            tunnel: [w633] -> w625
            tunnel: w612 -> [w631]
            n320 = timed-flat-sequence {
              tunnel: w651 -> [w657]
              tunnel: w652 -> [w658]
              tunnel: [w655] -> w647
              tunnel: [w658] -> w646
              tunnel: [w657] -> w645
              tunnel: [w656] -> w644
              tunnel: w650 -> [w655]
              tunnel: [w654] -> w642
              tunnel: w649 -> [w654]
              tunnel: [w653] -> w641
              tunnel: w648 -> [w653]
              tunnel: [w671] -> w640
              tunnel: [w668] -> w638
              tunnel: w647 -> [w663]
              tunnel: w646 -> [w670]
              tunnel: w645 -> [w669]
              tunnel: [w667] -> w636
              tunnel: w644 -> [w667]
              tunnel: [w666] -> w632
              tunnel: w643 -> [w665]
              tunnel: w642 -> [w664]
              tunnel: w641 -> [w662]
              tunnel: w631 -> [w661]
              tunnel: [w733] -> w637
              tunnel: [w734] -> w639
              tunnel: w640 -> [w734]
              tunnel: w638 -> [w733]
              tunnel: w636 -> [w729]
              tunnel: w635 -> [w728]
              tunnel: [w727] -> w634
              tunnel: [w726] -> w633
              tunnel: w632 -> [w726]
              frame #0 {
                n321 = node-c288() -> ()  [unwired: 1 in, 1 out]
                n322 = node-c288() -> ()  [unwired: 1 in, 1 out]
                n323 = Tick Count (ms)() -> (millisecond timer value=w656:u32)
              }
              frame #1 {
                n324 = node-c288() -> ()  [unwired: 1 in, 1 out]
                n325 = while {
                  tunnel: [w685] -> w671
                  tunnel: w669 -> [w683]
                  tunnel: [w681] -> w666
                  tunnel: w665 -> [w680]
                  tunnel: w664 -> [w679]
                  tunnel: w663 -> [w678]
                  tunnel: w662 -> [w677]
                  shift-right: [w682] -> w668
                  shift-left: w670 -> [w684]
                  tunnel: w661 -> [w674]
                  stop <- TRUE stop-if-true
                  # "Receive data is organised as:\nDate Time so2 DATA -1\nDate Time pmt voltage DATA 0\nDate Time lamp voltage DATA 1\nDate Time so2 DATA -1\nDate Time lamp int DATA 2\nDate Time internal temp DATA 3\nDate Time so2 DATA -1\nDate Time react temp DATA 4\nDate Time pres DATA 5\nDate Time so2 DATA -1\nDate Time flow DATA 6\nDate Time flags DATA 7\n\nDate Time Read Error -2"
                  n326 = for {
                    tunnel: w679 -> [w702]
                    tunnel: [w703] -> w685
                    tunnel: w683 -> [w700] mode=indexing
                    tunnel: [w704] -> w681
                    tunnel: w680 -> [w710]
                    tunnel: w678 -> [w705]
                    tunnel: w677 -> [w699]
                    shift-right: [w714] -> w682
                    shift-left: w684 -> [w715]
                    tunnel: w674 -> [w688]
                    i -> [w692]
                    # "Acquire every 330msec for 3 times\nto make 1 second"
                    # "SO2 Acquisition Loop"
                    n327 = call "Wait"("Count(mSec)"=w688) -> ()  [unwired: 1 out]
                    n328 = Concatenate Strings("ID", w700, "\r") -> (w698:string)
                    "Command In" <- w698
                    n329 = call "SO2 Serial Packet Write.vi"("VISA resource name In"=w705, "Data in"=w698, "error in (no error)"=w702) -> ("VISA resource name Out"=w707:refnum<visa-resource-name>, "error out"=w706:errorcluster)  [unwired: 11 in]
                    n330 = call "SO2 Serial Packet Read.vi"("VISA resource In"=w707, "error in"=w706) -> ("VISA resource Out"=w704:refnum<visa-resource-name>, "Data Out"=w695:string, "error out"=w703:errorcluster)  [unwired: 11 in]
                    "RAW DATA" <- w695
                    n331 = Equal?(x=w695, y="Read Error") -> (x = y?=w693:bool)
                    n332 = Get Date/Time In Seconds() -> (seconds since 1Jan1904=w687:timestamp)
                    n333 = case shown="False" w693 {
                      tunnel: [w718 "-2"] -> w708
                      tunnel: w692 -> [w717 _]
                      tunnel: w699 -> [w716 _]
                      frame False {
                        n334 = case shown="0" w717 {
                          tunnel: ["-1" w722 w724] -> w718
                          tunnel: w716 -> [_ w720 w723]
                          frame 0 {
                            # "Make internal flag\n-1 represent so2 data"
                          }
                          frame 2 {
                            # "Make internal flag"
                            n335 = Increment(x=w720) -> (x+1=w721:i32)
                            n336 = Number To Decimal String(number=w721) -> (decimal integer string=w722:string)  [unwired: 1 in]
                          }
                          frame 1, Default {
                            # "Make internal flag"
                            n337 = Number To Decimal String(number=w723) -> (decimal integer string=w724:string)  [unwired: 1 in]
                          }
                        }
                      }
                      frame True {
                      }
                    }
                    n338 = Increment(x=w715) -> (x+1=w711:i32)
                    n339 = Unbundle(w703) -> ("status"=w712:bool)  [unwired: 2 out]
                    n340 = call <vilib>:"Trim Whitespace.vi"("string"=w695) -> ("trimmed string"=w709:string)  [unwired: 1 in]
                    n341 = To Unsigned Long Integer(number=w687) -> (unsigned 32bit integer=w691:u32)
                    n342 = Subtract(x=w691, y=u32 2082844800) -> (x-y=w686:u32)
                    n343 = Select(t=w711, s=w712, f=w715) -> (s? t:f=w714:i32)
                    n344 = call <vilib>:"Space Constant.vi"() -> ("String"=w696:string)
                    n345 = Number To Decimal String(number=w686) -> (decimal integer string=w689:string)  [unwired: 1 in]
                    n346 = Build Array(w689, w696, w709, w696, w708) -> (w697:string[])
                    n347 = Enqueue Element(queue=w710, element=w697) -> ()  [unwired: 2 in, 3 out]
                  }
                  "Number of Send & Read Error\nfrom Acquire Loop" <- w682
                  n348 = call "Wait Until Next Multiple"("Count(mSec)"=u32 1000) -> ()  [unwired: 1 out]
                }
                n349 = node-c288() -> ()  [unwired: 1 in, 1 out]
              }
              frame #2 {
                n350 = node-c288() -> ()  [unwired: 1 in, 1 out]
                n351 = Tick Count (ms)() -> (millisecond timer value=w732:u32)
                n352 = Subtract(x=w732, y=w729) -> (x-y=w731:u32)
                "Acq Time" <- w731
                "Time taken history" <- w731
                n353 = Greater?(x=w731, y=w728) -> (0:w730:bool)
                n354 = Select(t=w731, s=w730, f=w728) -> (s? t:f=w727:u32)
                "Max Acq Time diff" <- w727
                n355 = node-c288() -> ()  [unwired: 1 in, 1 out]
              }
            }
          }
          n356 = node-c288(w613) -> ()  [unwired: 1 out]
        }
      }
      n357 = node-c288(w85) -> ()  [unwired: 1 out]
      n358 = node-c288(w83) -> ()  [unwired: 1 out]
      n359 = while {
        stop <- FALSE stop-if-true
        # "CAL MFC 3 status & control"
        n360 = Wait (ms)(milliseconds to wait=u32 1000) -> ()  [unwired: 1 out]
        n361 = call-poly "VISA Configure Serial Port"("VISA resource name"="VISA resource name 2", "timeout (10sec)"="timeout (10sec) 2", "termination char\n(0xA = '\\n' = LF)"=u8 13 ("termination char\n(0xA = '\\n' = LF)"), "Enable Termination\nChar (T)"=TRUE ("Enable Termination\nChar (T)"), "baud rate (9600)"=u32 19200) -> ("VISA resource name out"=w355:refnum<visa-resource-name>, "error out"=w351:errorcluster)  [unwired: 9 in]
        n362 = case shown="No Error" w351 {
          selector: w351 -> [w362 w412]
          tunnel: w355 -> [w363 w413]
          tunnel: [w361 w413] -> w354
          tunnel: [w360 w412] -> w353
          frame No Error {
            n363 = node-c288() -> (w358:T4)  [unwired: 4 in]
            n364 = timed-loop {
              tunnel: w363 -> [w386]
              tunnel: w362 -> [w384]
              tunnel: [w377] -> w361
              tunnel: [w372] -> w360
              shift-right: [w373] -> _
              shift-left: FALSE -> [w376]
              timing: w358 -> [_]
              timing-out: [_] -> w357
              shift-right: [w364] -> _
              shift-left: 0.0 -> [w366]
              stop <- w372 stop-if-true
              n365 = node-c288() -> ()  [unwired: 1 in, 1 out]
              n366 = local read "MFC_3 SLPM set value"() -> (w364:dbl)
              n367 = Not Equal?(x=w364, y=w366) -> (x != y?=w365:bool)
              n368 = case shown="True" w365 {
                tunnel: w386 -> [w394 w409]
                tunnel: [w394 w409] -> w385
                tunnel: w384 -> [w393 w408]
                tunnel: [w393 w408] -> w383
                tunnel: "A" -> [w397 w401]
                tunnel: [w395 w398] -> w381
                frame False {
                  n369 = Concatenate Strings(w397, "\r") -> (w395:string)
                }
                frame True {
                  n370 = Multiply(x="MFC_3 SLPM set value", y=u32 64000) -> (x*y=w405:dbl)
                  n371 = Divide(x=w405, y=u32 5) -> (x/y=w403:dbl)
                  n372 = To Unsigned Long Integer(number=w403) -> (unsigned 32bit integer=w402:u32)
                  n373 = Number To Decimal String(number=w402) -> (decimal integer string=w400:string)  [unwired: 1 in]
                  n374 = Concatenate Strings(w401, w400, "\r") -> (w398:string)
                }
              }
              n375 = VISA Flush I/O Buffer(VISA resource name=w385, error in (no error)=w383) -> (VISA resource name out=w388:refnum<visa-resource-name>, error out=w387:errorcluster)  [unwired: 1 in]
              n376 = Select(t=FALSE, s=w376, f=TRUE) -> (s? t:f=w373:bool)
              "status" <- w373
              n377 = VISA Write(VISA resource name=w388, write buffer=w381, error in (no error)=w387) -> (VISA resource name out=w380:refnum<visa-resource-name>, error out=w379:errorcluster)  [unwired: 1 out]
              n378 = VISA Flush I/O Buffer(VISA resource name=w380, error in (no error)=w379) -> (VISA resource name out=w390:refnum<visa-resource-name>, error out=w389:errorcluster)  [unwired: 1 in]
              n379 = VISA Read(VISA resource name=w390, byte count=u32 50, error in (no error)=w389) -> (VISA resource name out=w377:refnum<visa-resource-name>, read buffer=w371:string, error out=w372:errorcluster)  [unwired: 1 out]
              "Value Read 3" <- w371
              n380 = call <vilib>:"Space Constant.vi"() -> ("String"=w370:string)
              n381 = Spreadsheet String To Array(delimiter (Tab)=w370, format string="%f", spreadsheet string=w371, array type (2D Dbl)=dbl[] []) -> (array=→"MFC 3":dbl[])
              n382 = node-c288() -> ()  [unwired: 1 in, 1 out]
            }
            n383 = node-c288(w357) -> ()  [unwired: 1 out]
          }
          frame Error {
          }
        }
        n384 = VISA Close(VISA resource name=w354, error in (no error)=w353) -> (error out=→"error out 3":errorcluster)
      }
      n385 = while {
        stop <- FALSE stop-if-true
        # "CAL MFC 2 status & control"
        n386 = Wait (ms)(milliseconds to wait=u32 1000) -> ()  [unwired: 1 out]
        n387 = call-poly "VISA Configure Serial Port"("VISA resource name"="VISA resource name 3", "timeout (10sec)"="timeout (10sec) 3", "termination char\n(0xA = '\\n' = LF)"=u8 13 ("termination char\n(0xA = '\\n' = LF)"), "Enable Termination\nChar (T)"=TRUE ("Enable Termination\nChar (T)"), "baud rate (9600)"=u32 19200) -> ("VISA resource name out"=w285:refnum<visa-resource-name>, "error out"=w281:errorcluster)  [unwired: 9 in]
        n388 = case shown="No Error" w281 {
          selector: w281 -> [w292 w342]
          tunnel: w285 -> [w293 w343]
          tunnel: [w291 w343] -> w284
          tunnel: [w290 w342] -> w283
          frame No Error {
            n389 = node-c288() -> (w288:T4)  [unwired: 4 in]
            n390 = timed-loop {
              tunnel: w293 -> [w316]
              tunnel: w292 -> [w314]
              tunnel: [w307] -> w291
              tunnel: [w302] -> w290
              shift-right: [w303] -> _
              shift-left: FALSE -> [w306]
              timing: w288 -> [_]
              timing-out: [_] -> w287
              shift-right: [w294] -> _
              shift-left: 0.0 -> [w296]
              stop <- w302 stop-if-true
              n391 = node-c288() -> ()  [unwired: 1 in, 1 out]
              n392 = local read "MFC_2 SLPM set value"() -> (w294:dbl)
              n393 = Not Equal?(x=w294, y=w296) -> (x != y?=w295:bool)
              n394 = case shown="True" w295 {
                tunnel: w316 -> [w324 w339]
                tunnel: [w324 w339] -> w315
                tunnel: w314 -> [w323 w338]
                tunnel: [w323 w338] -> w313
                tunnel: "A" -> [w327 w331]
                tunnel: [w325 w328] -> w311
                frame False {
                  n395 = Concatenate Strings(w327, "\r") -> (w325:string)
                }
                frame True {
                  n396 = Multiply(x="MFC_2 SLPM set value", y=u32 64000) -> (x*y=w335:dbl)
                  n397 = Divide(x=w335, y=u32 5) -> (x/y=w333:dbl)
                  n398 = To Unsigned Long Integer(number=w333) -> (unsigned 32bit integer=w332:u32)
                  n399 = Number To Decimal String(number=w332) -> (decimal integer string=w330:string)  [unwired: 1 in]
                  n400 = Concatenate Strings(w331, w330, "\r") -> (w328:string)
                }
              }
              n401 = Select(t=FALSE, s=w306, f=TRUE) -> (s? t:f=w303:bool)
              "status 2" <- w303
              n402 = VISA Flush I/O Buffer(VISA resource name=w315, error in (no error)=w313) -> (VISA resource name out=w318:refnum<visa-resource-name>, error out=w317:errorcluster)  [unwired: 1 in]
              n403 = VISA Write(VISA resource name=w318, write buffer=w311, error in (no error)=w317) -> (VISA resource name out=w310:refnum<visa-resource-name>, error out=w309:errorcluster)  [unwired: 1 out]
              n404 = VISA Flush I/O Buffer(VISA resource name=w310, error in (no error)=w309) -> (VISA resource name out=w320:refnum<visa-resource-name>, error out=w319:errorcluster)  [unwired: 1 in]
              n405 = VISA Read(VISA resource name=w320, byte count=u32 50, error in (no error)=w319) -> (VISA resource name out=w307:refnum<visa-resource-name>, read buffer=w301:string, error out=w302:errorcluster)  [unwired: 1 out]
              "Value Read 2" <- w301
              n406 = call <vilib>:"Space Constant.vi"() -> ("String"=w300:string)
              n407 = Spreadsheet String To Array(delimiter (Tab)=w300, format string="%f", spreadsheet string=w301, array type (2D Dbl)=dbl[] []) -> (array=→"MFC 2":dbl[])
              n408 = node-c288() -> ()  [unwired: 1 in, 1 out]
            }
            n409 = node-c288(w287) -> ()  [unwired: 1 out]
          }
          frame Error {
          }
        }
        n410 = VISA Close(VISA resource name=w284, error in (no error)=w283) -> (error out=→"error out 2":errorcluster)
      }
      n411 = node-c288(w109) -> ()  [unwired: 1 out]
      n412 = while {
        stop <- FALSE stop-if-true
        n413 = node-c288() -> (w114:T4)  [unwired: 4 in]
        n414 = Create Network Stream Reader Endpoint(7:10 ("reader buffer size"), 9:T3 {"Message"="", "Message Data"=variant} ("Message Cluster"), 11:"/command/reader/SO2" ("reader url")) -> (0:w120:errorcluster, 3:w121:refnum<k21>)  [unwired: 4 in]
        n415 = timed-loop "Host->Target Command Reader" {
          shift-right: [w131] -> w118
          shift-left: w120 -> [w134]
          shift-right: [w132] -> w117
          shift-left: w121 -> [w133]
          tunnel: [TRUE] -> _
          timing: w114 -> [_]
          timing-out: [_] -> w113
          stop <- w125 stop-if-true
          # "Receive Commands from Host VI"
          n416 = node-c288() -> ()  [unwired: 1 in, 1 out]
          n417 = shared-variable-read(w133, w134) -> (w132:refnum<k21>, w127:errorcluster, w129:bool, w130:T3)  [unwired: 1 in]
          n418 = Or(x=w129, y=w127) -> (x .or. y?=w128:bool)
          n419 = case shown="False" w128 {
            selector: w128 -> [_ w270]
            tunnel: w127 -> [w142 w271]
            tunnel: [w141 w271] -> w131
            tunnel: w130 -> [w139 _]
            tunnel: [w140 w270] -> w125
            frame False {
              n420 = Unbundle By Name(w139) -> ("Message"=w138:string, "Message Data"=w137:variant)
              n421 = case shown="\"zeroing_interval\"" w138 {
                tunnel: w142 -> [w144 w149 w154 w159 w164 w169 w174 w179 w184 w189 w194 w199 w204 w209 w214 w219 w224 w229 w234 w239 w244 w249 w254 w258 w263 w268]
                tunnel: [w144 w148 w153 w158 w163 w168 w173 w178 w183 w188 w193 w198 w203 w208 w213 w218 w223 w228 w233 w238 w243 w248 w253 w256 w261 w266] -> w141
                tunnel: w137 -> [_ w147 w152 w157 w162 w167 w172 w177 w182 w187 w192 w197 w202 w207 w212 w217 w222 w227 w232 w237 w242 w247 w252 w259 w264 w269]
                tunnel: [TRUE _ _ _ _ _ _ _ _ _ _ _ _ _ _ _ _ _ _ _ _ _ _ _ _ _] -> w140
                frame "Stop", Default {
                }
                frame "V9" {
                  n422 = Variant To Data(error in=w149, type=FALSE, Variant=w147) -> (data=w145:bool, error out=w148:errorcluster)
                  "V9" <- w145
                  n423 = shared-variable "NI-cRIO9022-019C2C95\\Mod6\\DO7"(w145) -> ()  [unwired: 1 in, 1 out]
                }
                frame "MFC_2" {
                  n424 = Variant To Data(error in=w154, type=0.0, Variant=w152) -> (data=w150:dbl, error out=w153:errorcluster)
                  n425 = local write "MFC_2 SLPM set value"(w150) -> ()
                }
                frame "cal_gas_cylin_conc" {
                  n426 = Variant To Data(error in=w159, type=0.0, Variant=w157) -> (data=→"cal gas cylinder conc":dbl, error out=w158:errorcluster)
                }
                frame "sim_MOCCA_conc" {
                  n427 = Variant To Data(error in=w164, type=0.0, Variant=w162) -> (data=→"Simulate MOCCA Conc":dbl, error out=w163:errorcluster)
                }
                frame "Auto_zero" {
                  n428 = Variant To Data(error in=w169, type=FALSE, Variant=w167) -> (data=→"Auto Zeroing":bool, error out=w168:errorcluster)
                }
                frame "zeroing_interval" {
                  n429 = Variant To Data(error in=w174, type=0, Variant=w172) -> (data=→"ev8 zero interval":i32, error out=w173:errorcluster)
                }
                frame "MOCCA_window_delay_time" {
                  n430 = Variant To Data(error in=w179, type=0, Variant=w177) -> (data=→"MOCCA window delay time (sec)":i32, error out=w178:errorcluster)
                }
                frame "MOCCA_limit" {
                  n431 = Variant To Data(error in=w184, type=0, Variant=w182) -> (data=→"MOCCA SO2 Limit":i32, error out=w183:errorcluster)
                }
                frame "eV8_user_set_time" {
                  n432 = Variant To Data(error in=w189, type=0, Variant=w187) -> (data=→"ev8 user set time":i32, error out=w188:errorcluster)
                }
                frame "MFC_3" {
                  n433 = Variant To Data(error in=w194, type=0.0, Variant=w192) -> (data=w190:dbl, error out=w193:errorcluster)
                  n434 = local write "MFC_3 SLPM set value"(w190) -> ()
                }
                frame "Simulate STEL Conc" {
                  n435 = Variant To Data(error in=w199, type=0.0, Variant=w197) -> (data=→"Simulate STEL Conc":dbl, error out=w198:errorcluster)
                }
                frame "Simulate TWA Conc" {
                  n436 = Variant To Data(error in=w204, type=0.0, Variant=w202) -> (data=→"Simulate TWA Conc":dbl, error out=w203:errorcluster)
                }
                frame "Offset" {
                  n437 = Variant To Data(error in=w209, type=0.0, Variant=w207) -> (data=→"Zero":dbl, error out=w208:errorcluster)
                }
                frame "10mins STEL Limit" {
                  n438 = Variant To Data(error in=w214, type=0, Variant=w212) -> (data=→"10mins_STEL_limit":i32, error out=w213:errorcluster)
                }
                frame "UDP Time Offset" {
                  n439 = Variant To Data(error in=w219, type=0, Variant=w217) -> (data=→"UDP Time Stamp Offset":i32, error out=w218:errorcluster)
                }
                frame "8hr TWA Limit" {
                  n440 = Variant To Data(error in=w224, type=0, Variant=w222) -> (data=→"8hr_TWA_limit":i32, error out=w223:errorcluster)
                }
                frame "Slope" {
                  n441 = Variant To Data(error in=w229, type=0.0, Variant=w227) -> (data=→"Slope":dbl, error out=w228:errorcluster)
                }
                frame "V8" {
                  n442 = Variant To Data(error in=w234, type=FALSE, Variant=w232) -> (data=w230:bool, error out=w233:errorcluster)
                  "V8" <- w230
                  n443 = shared-variable "NI-cRIO9022-019C2C95\\Mod6\\DO6"(w230) -> ()  [unwired: 1 in, 1 out]
                }
                frame "Stop File Write" {
                  n444 = Variant To Data(error in=w239, type=FALSE, Variant=w237) -> (data=→"Stop File Write":bool, error out=w238:errorcluster)
                }
                frame "SO2_MOCCA_Alarm" {
                  n445 = Variant To Data(error in=w244, type=FALSE, Variant=w242) -> (data=→"SO2 Inflight MOCCA Alarm\n(default = OFF)":bool, error out=w243:errorcluster)
                }
                frame "Flight Number" {
                  n446 = Variant To Data(error in=w249, type="", Variant=w247) -> (data=→"Flight Number":string, error out=w248:errorcluster)
                }
                frame "V6" {
                  n447 = Variant To Data(error in=w254, type=FALSE, Variant=w252) -> (data=w250:bool, error out=w253:errorcluster)
                  "V6" <- w250
                  n448 = shared-variable "NI-cRIO9022-019C2C95\\Mod6\\DO4"(w250) -> ()  [unwired: 1 in, 1 out]
                }
                frame "Simulate Conc" {
                  n449 = Variant To Data(error in=w258, type=FALSE, Variant=w259) -> (data=→"Simulate\nconc":bool, error out=w256:errorcluster)
                }
                frame "calcon_save" {
                  n450 = Variant To Data(error in=w263, type=FALSE, Variant=w264) -> (data=→"calcon save to file":bool, error out=w261:errorcluster)
                }
                frame "mean_cal_status" {
                  n451 = Variant To Data(error in=w268, type=FALSE, Variant=w269) -> (data=→"Mean Cal\n(default = ON)":bool, error out=w266:errorcluster)
                }
              }
            }
            frame True {
            }
          }
          n452 = node-c288() -> ()  [unwired: 1 in, 1 out]
        }
        n453 = node-c288(w113) -> ()  [unwired: 1 out]
        n454 = Destroy Stream Endpoint(8:w118, 11:w117) -> (0:→"error out 4":errorcluster)
        n455 = Wait (ms)(milliseconds to wait=u32 1000) -> ()  [unwired: 1 out]
      }
      n456 = while {
        tunnel: w96 -> [w497]
        stop <- w498 stop-if-true
        # "UDP Broadcast loop"
        # "Broadcast UDP SO2 Data"
        n457 = node-c288() -> (w500:T4)  [unwired: 4 in]
        n458 = String To IP(1:"239.1.4.6" ("name")) -> (0:w502:u32)
        n459 = call-poly <vilib>:"UDP Multicast Open.vi"("time-to-live (1)"=u16 5, "port"=u16 10001) -> ("error out"=w510:errorcluster, "connection ID"=w511:refnum<k16>)  [unwired: 8 in]
        n460 = timed-loop {
          tunnel: w511 -> [w531]
          tunnel: w510 -> [w530]
          tunnel: [w517] -> w506
          shift-right: [w520] -> _
          shift-left: FALSE -> [w523]
          tunnel: [w515] -> w504
          tunnel: w502 -> [w519]
          tunnel: u16 50001 ("port or service name") -> [w518]
          timing: w500 -> [_]
          timing-out: [_] -> w499
          tunnel: [w513] -> w498
          tunnel: w497 -> [w512]
          stop <- w514 stop-if-true
          n461 = node-c288() -> ()  [unwired: 1 in, 1 out]
          n462 = local read "Flight Number"() -> (w526:string)
          n463 = Select(t=FALSE, s=w523, f=TRUE) -> (s? t:f=w520:bool)
          "UDP packet \nstatus" <- w520
          n464 = feedback-in #2(w526) -> ()
          n465 = feedback #2() -> (w525:string)  [unwired: 1 in]
          n466 = Not Equal?(x=w526, y=w525) -> (x != y?=w524:bool)
          n467 = flat-sequence {
            tunnel: w519 -> [w539]
            tunnel: w530 -> [w540]
            tunnel: w531 -> [w541]
            tunnel: [w541] -> w529
            tunnel: [w540] -> w528
            tunnel: [w539] -> w527
            tunnel: w524 -> [w538]
            tunnel: w518 -> [w551]
            tunnel: w529 -> [w550]
            tunnel: w528 -> [w549]
            tunnel: w527 -> [w548]
            tunnel: [w547] -> w517
            tunnel: [w546] -> w515
            tunnel: w512 -> [w545]
            frame #0 {
              n468 = feedback #3(u32 0) -> (w535:u32)
              n469 = case shown="True" w538 {
                tunnel: w535 -> [w542 _]
                tunnel: [w542 u32 0] -> w534
                frame False {
                }
                frame True {
                }
              }
              "UDP_Pack_num" <- w534
              n470 = Increment(x=w534) -> (x+1=w536:u32)
              n471 = feedback-in #3(w536) -> ()
            }
            frame #1 {
              n472 = Dequeue Element(queue=w545) -> (element=w544:string)  [unwired: 2 in, 3 out]
              n473 = UDP Write(address=w548, port or service name=w551, connection ID=w550, data in=w544, 8:w549) -> (error out=w546:errorcluster, 3:w547:refnum<k16>)  [unwired: 1 in]
            }
          }
          n474 = local read "stop"() -> (w513:bool)
          n475 = Unbundle(w515) -> ("status"=w516:bool)  [unwired: 2 out]
          n476 = node-c288() -> ()  [unwired: 1 in, 1 out]
          n477 = Compound Arithmetic op=OR(w516, w513) -> (w514:bool)
        }
        n478 = node-c288(w499) -> ()  [unwired: 1 out]
        n479 = UDP Close(connection ID=w506, 8:w504) -> (error out=→"UDP_Out_Error":errorcluster)  [unwired: 1 out]
        n480 = Wait (ms)(milliseconds to wait=u32 1000) -> ()  [unwired: 1 out]
      }
      n481 = while {
        tunnel: w94 -> [w456]
        tunnel: w95 -> [w455]
        stop <- w459 stop-if-true
        # "TCP Loop writing to SEPTIC Tank"
        n482 = TCP Open Connection(address="192.168.101.108", remote port or service name=u16 3502) -> (connection ID=w462:refnum<k5>, error out=w457:errorcluster)  [unwired: 3 in]
        n483 = case shown="No Error" w457 {
          selector: w457 -> [w467 w494]
          tunnel: w462 -> [w472 w495]
          tunnel: [w471 w495] -> w461
          tunnel: [w470 w494] -> w460
          tunnel: [w469 w493] -> w459
          tunnel: w455 -> [w466 _]
          tunnel: w456 -> [w465 _]
          frame No Error {
            n484 = node-c288() -> (w474:T4)  [unwired: 4 in]
            n485 = timed-loop {
              tunnel: w472 -> [w488]
              tunnel: w467 -> [w487]
              tunnel: [w486] -> w471
              tunnel: [w485] -> w470
              tunnel: [w475] -> w469
              shift-right: [w479] -> _
              shift-left: FALSE -> [w482]
              timing: w474 -> [_]
              timing-out: [_] -> w473
              tunnel: w466 -> [w478]
              tunnel: w465 -> [w477]
              stop <- w483 stop-if-true
              n486 = node-c288() -> ()  [unwired: 1 in, 1 out]
              n487 = Dequeue Element(queue=w478, error in (no error)=w477) -> (element=w476:string)  [unwired: 1 in, 3 out]
              n488 = Select(t=FALSE, s=w482, f=TRUE) -> (s? t:f=w479:bool)
              "TCP packet\nSend to SEPTIC" <- w479
              n489 = TCP Write(connection ID=w488, data in=w476, error in (no error)=w487) -> (connection ID out=w486:refnum<k5>, error out=w485:errorcluster)  [unwired: 1 in, 1 out]
              n490 = local read "stop"() -> (w475:bool)
              n491 = Unbundle(w485) -> ("status"=w484:bool)  [unwired: 2 out]
              n492 = node-c288() -> ()  [unwired: 1 in, 1 out]
              n493 = Compound Arithmetic op=OR(w484, w475) -> (w483:bool)
            }
            n494 = node-c288(w473) -> ()  [unwired: 1 out]
          }
          frame Error {
            n495 = local read "stop"() -> (w493:bool)
          }
        }
        n496 = TCP Close Connection(connection ID=w461, error in (no error)=w460) -> (error out=→"SEPTIC TCP Error Out":errorcluster)  [unwired: 1 in, 1 out]
        n497 = Wait (ms)(milliseconds to wait=u32 1000) -> ()  [unwired: 1 out]
      }
      n498 = while {
        tunnel: w100 -> [w556]
        tunnel: w99 -> [w555]
        stop <- w559 stop-if-true
        # "TCP Loop writing to FISH Tank"
        n499 = TCP Open Connection(address="192.168.101.110", remote port or service name=u16 3502) -> (connection ID=w562:refnum<k5>, error out=w557:errorcluster)  [unwired: 3 in]
        n500 = case shown="No Error" w557 {
          selector: w557 -> [w567 w594]
          tunnel: w562 -> [w572 w595]
          tunnel: [w571 w595] -> w561
          tunnel: [w570 w594] -> w560
          tunnel: [w569 w593] -> w559
          tunnel: w556 -> [w566 _]
          tunnel: w555 -> [w565 _]
          frame No Error {
            n501 = node-c288() -> (w574:T4)  [unwired: 4 in]
            n502 = timed-loop {
              tunnel: w572 -> [w588]
              tunnel: w567 -> [w587]
              tunnel: [w586] -> w571
              tunnel: [w585] -> w570
              tunnel: [w582] -> w569
              shift-right: [w578] -> _
              shift-left: FALSE -> [w581]
              timing: w574 -> [_]
              timing-out: [_] -> w573
              tunnel: w566 -> [w577]
              tunnel: w565 -> [w576]
              stop <- w583 stop-if-true
              n503 = node-c288() -> ()  [unwired: 1 in, 1 out]
              n504 = Dequeue Element(queue=w577, error in (no error)=w576) -> (element=w575:string)  [unwired: 1 in, 3 out]
              n505 = Select(t=FALSE, s=w581, f=TRUE) -> (s? t:f=w578:bool)
              "TCP packet\nSend to FISH" <- w578
              n506 = TCP Write(connection ID=w588, data in=w575, error in (no error)=w587) -> (connection ID out=w586:refnum<k5>, error out=w585:errorcluster)  [unwired: 1 in, 1 out]
              n507 = local read "stop"() -> (w582:bool)
              n508 = Unbundle(w585) -> ("status"=w584:bool)  [unwired: 2 out]
              n509 = node-c288() -> ()  [unwired: 1 in, 1 out]
              n510 = Compound Arithmetic op=OR(w584, w582) -> (w583:bool)
            }
            n511 = node-c288(w573) -> ()  [unwired: 1 out]
          }
          frame Error {
            n512 = local read "stop"() -> (w593:bool)
          }
        }
        n513 = TCP Close Connection(connection ID=w561, error in (no error)=w560) -> (error out=→"FISH TCP Error Out":errorcluster)  [unwired: 1 in, 1 out]
        n514 = Wait (ms)(milliseconds to wait=u32 1000) -> ()  [unwired: 1 out]
      }
    }
    frame Error {
    }
  }
  n515 = VISA Close(VISA resource name=w36, error in (no error)=w35) -> (error out=→"Serial Visa Error":errorcluster)
